vi "Gas Rack Cal UI.vi"(11 "Calling VI Ref":refnum<vi>) -> ()   [LabVIEW 2013]
uses:
  Type Defs/Units Type Def (DAQ Rack).ctl
  Type Defs/Gas Rack Channel Type Def (RIO).ctl
  Type Defs/Targets Type Def.ctl
  Type Defs/Target Cluster Type Def.ctl
  Type Defs/Setpoint Cluster Type Def.ctl
  Type Defs/Rack Version Type Def.ctl
  Type Defs/Registered System.ctl
  Type Defs/System Type.ctl
  Type Defs/TCP Data Stream Mode (PC).ctl
  <vilib>/Utility/miscctls.llb/LVRowAndColumnTypeDef.ctl
  <vilib>/Utility/file.llb/Write To Spreadsheet File (string).vi
  <vilib>/Utility/file.llb/Read From Spreadsheet File (string).vi
  <userlib>/_OpenG.lib/array/array.llb/Remove Duplicates from 1D Array (DBL)__ogtk.vi
  <userlib>/_OpenG.lib/array/array.llb/Search 1D Array (String)__ogtk.vi
  <vilib>/ptbypt/NI_PtbyPt.lvlib
  <vilib>/Analysis/NI_AALPro.lvlib
  <resource>/objmgr/daqmx.rc
  <vilib>/Utility/config.llb/NI_LVConfig.lvlib
  <vilib>/FTP/NI_FTP.lvlib
panel:
  out "RIO Found":bool
  out "Lost Connection":bool
  in  "Stop Second Loop":bool
  out "a0":dbl format="%#.4g"
  out "a2":dbl format="%#.4g"
  out "a1":dbl format="%#.4g"
  out "a3":dbl format="%#.4g"
  out "a4":dbl format="%#.4g"
  in  "App Dir":path
  in  "Load Indicator Tab":enum32{"Page 1"}(tab)
  in  "Header Tab":enum32{"Page 1", "Page 2"}(tab)
  in  "Header OK":bool
  in  "Header Cancel":bool
  in  "Header Comments":string[][](table)=[[""], [""], [""]]
  in  "Cal Standards Table":string[][](table)=[["", ""], ["", ""], ["", ""], ["", ""], ["", ""]]
  in  "Sys Cal Table":string[][](table)=[["", ""], ["", ""], ["", ""], ["", ""], ["", ""]]
  in  "Header Table 1":string[][](table)=[[""], [""], [""], [""], [""], [""], [""], [""]]
  in  "Header Table 2":string[][](table)=[[""], [""], [""], [""], [""], [""], [""]]
  in  "debug":bool=TRUE
  in  "Output Tab":enum32{"Page 1", "Page 2"}(tab)
  out "Row":i32
  in  "Main Tab":enum32{"Page 1", "Page 2"}(tab)
  in  "Channel to Cal":T1
  in  "Transfer Cal":bool
  in  "Verify Tab":enum32{"Page 1", "Page 2"}(tab)
  out "Ver Reading":dbl=0.0016 caption="reading" format="%#.4g"
  in  "Hide Devs":bool
  in  "Auto":bool
  in  "Hide Cal Values":bool
  in  "Verify Edit":bool
  in  "Verify Table":string[][](table)=[["", "0", "0"], ["", "3", "3"], ["", "6", "6"], ["", "9", "9"], ["", "12", "12"], ["", "15", "15"], ["", "", ""], ["", "", ""], ["", "", ""], ["", "", ""]]
  in  "Verify Read":bool
  in  "ms":u32=1000
  in  "avg":i32=5
  in  "Save Cal":bool
  in  "Cancel Verify":bool
  in  "Cal Tab":enum32{"Apply", "Cal"}(tab)
  in  "Cancel Cal":bool
  in  "Apply Cal":bool
  in  "Confirm Cal Point":bool
  in  "Master Value":dbl caption="cal pt" format="%#.4g"
  out "Cal Reading":dbl=0.0016 caption="reading" format="%#.4g"
  in  "4th Point Cal":bool
  out "Reading Value 4":dbl caption="reading" format="%#.4g"
  in  "Cal Value 4":dbl caption="cal pt" format="%#.4g"
  in  "5th Point Cal":bool
  out "Reading Value 5":dbl caption="reading" format="%#.4g"
  in  "Cal Value 5":dbl caption="cal pt" format="%#.4g"
  in  "Start Verification":bool
  in  "Header":bool
  out "Cal Table":string[][](table)=[["AI-00", "V", "", "", "", "", "", "", "", "", "", "", "", "", "", "", "", "", "", "", "", "", "", "", "", "", "", "", "", "", "", ""], ["AI-01", "V", "", "", "", "", "", "", "", "", "", "", "", "", "", "", "", "", "", "", "", "", "", "", "", "", "", "", "", "", "", ""], ["AI-02", "V", "", "", "", "", "", "", "", "", "", "", "", "", "", "", "", "", "", "", "", "", "", "", "", "", "", "", "", "", "", ""], ["AI-03", "V", "", "", "", "", "", "", "", "", "", "", "", "", "", "", "", "", "", "", "", "", "", "", "", "", "", "", "", "", "", ""], ["AI-04", "V", "", "", "", "", "", "", "", "", "", "", "", "", "", "", "", "", "", "", "", "", "", "", "", "", "", "", "", "", "", ""], ["AI-05", "V", "", "", "", "", "", "", "", "", "", "", "", "", "", "", "", "", "", "", "", "", "", "", "", "", "", "", "", "", "", ""], ["AI-06", "V", "", "", "", "", "", "", "", "", "", "", "", "", "", "", "", "", "", "", "", "", "", "", "", "", "", "", "", "", "", ""], ["AI-07", "V", "", "", "", "", "", "", "", "", "", "", "", "", "", "", "", "", "", "", "", "", "", "", "", "", "", "", "", "", "", ""], ["AI-08", "V", "", "", "", "", "", "", "", "", "", "", "", "", "", "", "", "", "", "", "", "", "", "", "", "", "", "", "", "", "", ""], ["AI-09", "V", "", "", "", "", "", "", "", "", "", "", "", "", "", "", "", "", "", "", "", "", "", "", "", "", "", "", "", "", "", ""], ["AI-10", "V", "", "", "", "", "", "", "", "", "", "", "", "", "", "", "", "", "", "", "", "", "", "", "", "", "", "", "", "", "", ""], ["AI-11", "V", "", "", "", "", "", "", "", "", "", "", "", "", "", "", "", "", "", "", "", "", "", "", "", "", "", "", "", "", "", ""], ["AI-12", "V", "", "", "", "", "", "", "", "", "", "", "", "", "", "", "", "", "", "", "", "", "", "", "", "", "", "", "", "", "", ""], ["AI-13", "V", "", "", "", "", "", "", "", "", "", "", "", "", "", "", "", "", "", "", "", "", "", "", "", "", "", "", "", "", "", ""], ["AI-14", "V", "", "", "", "", "", "", "", "", "", "", "", "", "", "", "", "", "", "", "", "", "", "", "", "", "", "", "", "", "", ""], ["AI-15", "V", "", "", "", "", "", "", "", "", "", "", "", "", "", "", "", "", "", "", "", "", "", "", "", "", "", "", "", "", "", ""], ["AI-16", "V", "", "", "", "", "", "", "", "", "", "", "", "", "", "", "", "", "", "", "", "", "", "", "", "", "", "", "", "", "", ""], ["AI-17", "V", "", "", "", "", "", "", "", "", "", "", "", "", "", "", "", "", "", "", "", "", "", "", "", "", "", "", "", "", "", ""], ["AI-18", "V", "", "", "", "", "", "", "", "", "", "", "", "", "", "", "", "", "", "", "", "", "", "", "", "", "", "", "", "", "", ""], ["AI-19", "V", "", "", "", "", "", "", "", "", "", "", "", "", "", "", "", "", "", "", "", "", "", "", "", "", "", "", "", "", "", ""], ["AI-20", "V", "", "", "", "", "", "", "", "", "", "", "", "", "", "", "", "", "", "", "", "", "", "", "", "", "", "", "", "", "", ""], ["AI-21", "V", "", "", "", "", "", "", "", "", "", "", "", "", "", "", "", "", "", "", "", "", "", "", "", "", "", "", "", "", "", ""], ["AI-22", "V", "", "", "", "", "", "", "", "", "", "", "", "", "", "", "", "", "", "", "", "", "", "", "", "", "", "", "", "", "", ""], ["AI-23", "V", "", "", "", "", "", "", "", "", "", "", "", "", "", "", "", "", "", "", "", "", "", "", "", "", "", "", "", "", "", ""], ["AI-24", "V", "", "", "", "", "", "", "", "", "", "", "", "", "", "", "", "", "", "", "", "", "", "", "", "", "", "", "", "", "", ""], ["AI-25", "V", "", "", "", "", "", "", "", "", "", "", "", "", "", "", "", "", "", "", "", "", "", "", "", "", "", "", "", "", "", ""], ["AI-26", "V", "", "", "", "", "", "", "", "", "", "", "", "", "", "", "", "", "", "", "", "", "", "", "", "", "", "", "", "", "", ""], ["AI-27", "V", "", "", "", "", "", "", "", "", "", "", "", "", "", "", "", "", "", "", "", "", "", "", "", "", "", "", "", "", "", ""], ["AI-28", "V", "", "", "", "", "", "", "", "", "", "", "", "", "", "", "", "", "", "", "", "", "", "", "", "", "", "", "", "", "", ""], ["AI-29", "V", "", "", "", "", "", "", "", "", "", "", "", "", "", "", "", "", "", "", "", "", "", "", "", "", "", "", "", "", "", ""], ["AI-30", "V", "", "", "", "", "", "", "", "", "", "", "", "", "", "", "", "", "", "", "", "", "", "", "", "", "", "", "", "", "", ""], ["AI-31", "V", "", "", "", "", "", "", "", "", "", "", "", "", "", "", "", "", "", "", "", "", "", "", "", "", "", "", "", "", "", ""], ["TC-00", "degF", "", "", "", "", "", "", "", "", "", "", "", "", "", "", "", "", "", "", "", "", "", "", "", "", "", "", "", "", "", ""], ["TC-01", "degF", "", "", "", "", "", "", "", "", "", "", "", "", "", "", "", "", "", "", "", "", "", "", "", "", "", "", "", "", "", ""], ["TC-02", "degF", "", "", "", "", "", "", "", "", "", "", "", "", "", "", "", "", "", "", "", "", "", "", "", "", "", "", "", "", "", ""], ["TC-03", "degF", "", "", "", "", "", "", "", "", "", "", "", "", "", "", "", "", "", "", "", "", "", "", "", "", "", "", "", "", "", ""], ["TC-04", "degF", "", "", "", "", "", "", "", "", "", "", "", "", "", "", "", "", "", "", "", "", "", "", "", "", "", "", "", "", "", ""], ["TC-05", "degF", "", "", "", "", "", "", "", "", "", "", "", "", "", "", "", "", "", "", "", "", "", "", "", "", "", "", "", "", "", ""], ["TC-06", "degF", "", "", "", "", "", "", "", "", "", "", "", "", "", "", "", "", "", "", "", "", "", "", "", "", "", "", "", "", "", ""], ["TC-07", "degF", "", "", "", "", "", "", "", "", "", "", "", "", "", "", "", "", "", "", "", "", "", "", "", "", "", "", "", "", "", ""], ["TC-08", "degF", "", "", "", "", "", "", "", "", "", "", "", "", "", "", "", "", "", "", "", "", "", "", "", "", "", "", "", "", "", ""], ["TC-09", "degF", "", "", "", "", "", "", "", "", "", "", "", "", "", "", "", "", "", "", "", "", "", "", "", "", "", "", "", "", "", ""], ["TC-10", "degF", "", "", "", "", "", "", "", "", "", "", "", "", "", "", "", "", "", "", "", "", "", "", "", "", "", "", "", "", "", ""], ["TC-11", "degF", "", "", "", "", "", "", "", "", "", "", "", "", "", "", "", "", "", "", "", "", "", "", "", "", "", "", "", "", "", ""], ["TC-12", "degF", "", "", "", "", "", "", "", "", "", "", "", "", "", "", "", "", "", "", "", "", "", "", "", "", "", "", "", "", "", ""], ["TC-13", "degF", "", "", "", "", "", "", "", "", "", "", "", "", "", "", "", "", "", "", "", "", "", "", "", "", "", "", "", "", "", ""], ["TC-14", "degF", "", "", "", "", "", "", "", "", "", "", "", "", "", "", "", "", "", "", "", "", "", "", "", "", "", "", "", "", "", ""], ["TC-15", "degF", "", "", "", "", "", "", "", "", "", "", "", "", "", "", "", "", "", "", "", "", "", "", "", "", "", "", "", "", "", ""], ["", "", "", "", "", "", "", "", "", "", "", "", "", "", "", "", "", "", "", "", "", "", "", "", "", "", "", "", "", "", "", ""]]
  out "Tank IP:":string
  in  "Start Cal":bool
  in  "1st Point Cal":bool
  out "Reading Value 1":dbl caption="Read Data" format="%#.4g"
  in  "Cal Value 1":dbl caption="Cal Point" format="%#.4g"
  in  "2nd Point Cal":bool
  out "Reading Value 2":dbl caption="reading" format="%#.4g"
  in  "Cal Value 2":dbl caption="cal pt" format="%#.4g"
  in  "Cal Unit":T2
  in  "3rd Point Cal":bool
  out "Reading Value 3":dbl caption="reading" format="%#.4g"
  in  "Cal Value 3":dbl caption="cal pt" format="%#.4g"
  in  "View Spreadsheet":bool
  # "Channel Data"
  # "System Calibration Components"
  # "Calibration Standards Used"
  # "Output Control"
  # "Enter Header Info"
  # "Calibration"
  # "Verification"
  # "Select Channel to Calibrate"
  # "Cal Spreadsheet"
  # "*Excel must be closed to return control to this app."
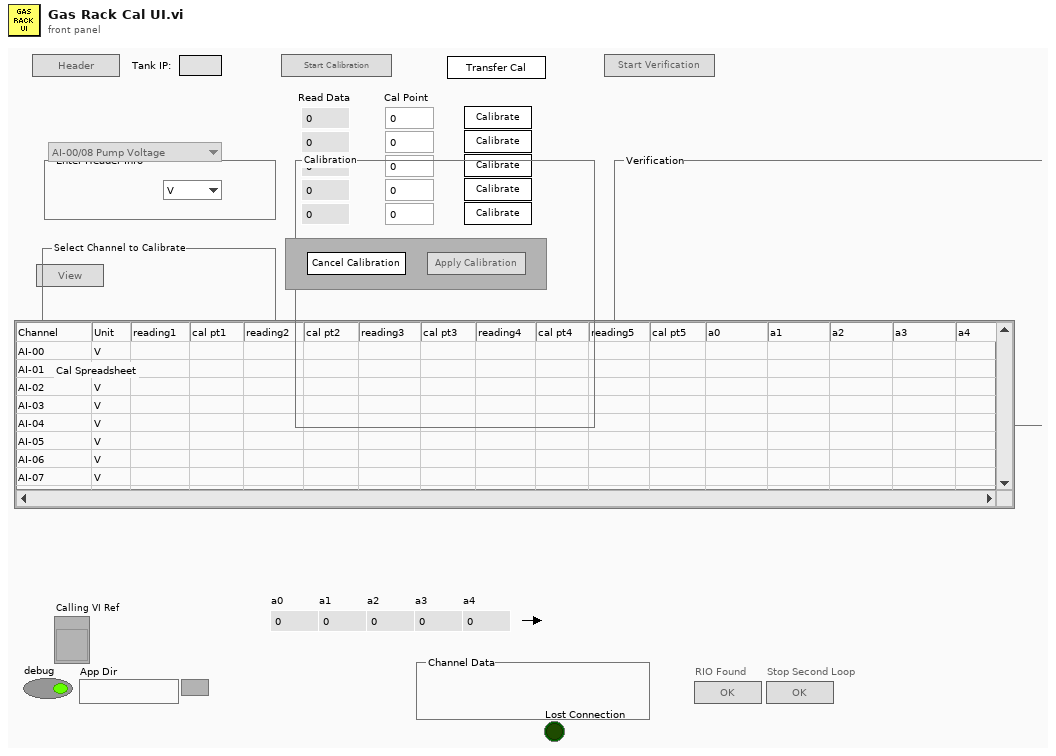
[diagram p1: front panel]
types:
  T1 = typedef "Gas Rack Channel Type Def (RIO).ctl" = enum16{"AI-00/08 Pump Voltage", "AI-01/09 Pump Current", "AI-02/10 Pressure", "AI-03/11 Flow", "AI-04/12 Controller Voltage", "AI-07/15 Controller Current", "AI-06/14 Temperature", "AI-05/13 Spare"}
  T2 = typedef "Units Type Def (DAQ Rack).ctl" = enum16{"V", "mA", "A", "Hz", "deg C"}
  T3 = typedef "Registered System.ctl" = cluster{"System Type":T4, "Serial Number":string, "ID":string, "Cal File?":bool}
  T4 = typedef "System Type.ctl" = enum16{"DAQ Rack", "DAQ Cart", "RIO", "cDAQ", "unknown", "open"}
  T5 = typedef "Rack Version Type Def.ctl" = enum16{"Volts & TC", "Volts", "RIO", "cDAQ", "Volts & Current", "Cart"}
  T6 = typedef "Targets Type Def.ctl" = cluster{"V Targets":T7, "5V Targets":T7, "mA Targets":T7, "A Targets":T7, "Hz Targets":T7, "TC Targets":T7, "V Setpoints":T8, "5V Setpoints":T8, "mA Setpoints ":T8, "A Setpoints":T8, "Hz Setpoints":T8, "25A Setpoints":T8, "25A Targets":T7, "CT Targets":T7, "DegC Targets":T7, "kPa Targets":T7, "LpH Targets":T7, "CT Setpoints":T8, "DegC Setpoints":T8, "kPa Setpoints":T8, "LpH Setpoints":T8}
  T7 = typedef "Target Cluster Type Def.ctl" = cluster{"target1":dbl, "target2":dbl, "target3":dbl, "target4":dbl, "target5":dbl, "target6":dbl, "target7":dbl, "target8":dbl, "target9":dbl, "target10":dbl}
  T8 = typedef "Setpoint Cluster Type Def.ctl" = cluster{"setpoint1":dbl, "setpoint2":dbl, "setpoint3":dbl, "setpoint4":dbl, "setpoint5":dbl}
  T9 = cluster{"Error":errorcluster, "Cal Log":string[][], "Cal Log Header":string[], "Cal Files Base Path":path, "Default Cal Log":string[][], "Samples to Avg":i32, "Base Path":path, "Cal Targets Path":path, "Calling VI Ref":refnum<vi>, "Selected Chassis":tag, "debug":bool, "Verify Table":string[][], "Cal Template Path":path, "Cal Spreadsheet Path":path, "Verify Table Ref":refnum<vi>, "Init Mean":bool, "Auto":bool, "App Dir":path, "DAQ Rack":string, "Cal File Path":path, "Targets":T6, "Cal Unit":T2, "Channel to Cal":T1, "Rack Version":T5, "Verification":bool, "Registered Systems":T3[], "Desired System":T3, "Cal Target Array":string[], "LastCalPt":i32, "StreamCtrlActive":bool}
  T10 = enum8{"Enabled", "Disabled", "Disabled and Grayed Out"}
  T11 = typedef "TCP Data Stream Mode (PC).ctl" = enum16{"Init", "Read Data", "Close"}
  T12 = typedef "LVRowAndColumnTypeDef.ctl" = cluster{"Row":i32, "Column":i32}
  T13 = enum32{"Bad", "Idle", "Run top level", "Running"}
  T14 = cluster{"[0]":dbl, "[1]":dbl, "[2]":dbl, "[3]":dbl, "[4]":dbl, "[5]":dbl, "[6]":dbl, "[7]":dbl, "[8]":dbl, "[9]":dbl}
  T15 = typedef "NI_LVConfig.lvlib/Config Data RefNum.ctl" = refnum<k1>
  T16 = typedef "New Channel Type Def (RIO).ctl" = enum16{"AI-00/08 Pos 1 Pump Voltage", "AI-01/09 Pos 2 Pump Voltage", "AI-02/10 Pos 3 Pump Voltage", "AI-03/11 Pos 4 Pump Voltage", "AI-04/12 Pos 5 Pump Voltage", "AI-05/13 Pos 6 Pump Voltage", "AI-06 Spare", "AI-14 Spare", "AI-07 Spare", "AI-15 Power Supply Voltage", "AI-16 Pos 1 Pump Current", "AI-17 Pos 2 Pump Current", "AI-18 Pos 3 Pump Current", "AI-19 Pos 4 Pump Current", "AI-20 Pos 5 Pump Current", "AI-21 Pos 6 Pump Current", "AI-16 Pos 1 Pump Speed", "AI-17 Pos 2 Pump Speed", "AI-18 Pos 3 Pump Speed", "AI-19 Pos 4 Pump Speed", "AI-20 Pos 5 Pump Speed", "AI-21 Pos 6 Pump Speed", "AI-22 Pos 1 Controller Current", "AI-23 Pos 2 Controller Current", "AI-24 Pos 3 Controller Current", "AI-25 Pos 4 Controller Current", "AI-26 Pos 5 Controller Current", "AI-27 Pos 6 Controller Current", "AI-28 Tank 1 Temperature", "AI-29 Tank 2 Temperature", "AI-30 Pos 1 Pump Pressure", "AI-31 Pos 2 Pump Pressure", "AI-32 Pos 3 Pump Pressure", "AI-33 Pos 4 Pump Pressure", "AI-34 Pos 5 Pump Pressure", "AI-35 Pos 6 Pump Pressure", "AI-36 Pos 1 Pump Flow", "AI-37 Pos 2 Pump Flow", "AI-38 Pos 3 Pump Flow", "AI-39 Pos 4 Pump Flow", "AI-40 Pos 5 Pump Flow", "AI-41 Pos 6 Pump Flow", "AI-42 Spare", "AI-43 Spare", "AI-44 Spare", "AI-45 Spare", "AI-46 Spare", "AI-47 Spare", "AI-00/08 Pos 1 Controller Voltage", "AI-01/09 Pos 2 Controller Voltage", "AI-02/10 Pos 3 Controller Voltage", "AI-03/11 Pos 4 Controller Voltage", "AI-04/12 Pos 5 Controller Voltage", "AI-05/13 Pos 6 Controller Voltage"}
  T17 = typedef "Rack Version Type Def.ctl" = enum16{"Volts & TC", "Volts", "RIO", "Volts & Current", "Cart"}
  T18 = typedef "Registered System.ctl" = cluster{"System Type":T19, "Serial Number":u32, "ID":string, "Cal File?":bool}
  T19 = typedef "System Type.ctl" = enum16{"DAQ Rack", "DAQ Cart", "RIO", "unknown", "open"}
  T20 = cluster{"Error":errorcluster, "Cal Log":string[][], "Cal Log Header":string[], "Cal Files Base Path":path, "Default Cal Log":string[][], "Samples to Avg":i32, "Base Path":path, "Cal Targets Path":path, "Calling VI Ref":refnum<vi>, "Selected Chassis":tag, "debug":bool, "Verify Table":string[][], "Cal Template Path":path, "Cal Spreadsheet Path":path, "Verify Table Ref":refnum<vi>, "Init Mean":bool, "Auto":bool, "App Dir":path, "DAQ Rack":string, "Cal File Path":path, "Targets":T6, "Cal Unit":T2, "Channel to Cal":T16, "Rack Version":T17, "Verification":bool, "Registered Systems":T18[], "Desired System":T18, "Cal Target Array":string[], "LastCalPt":i32}
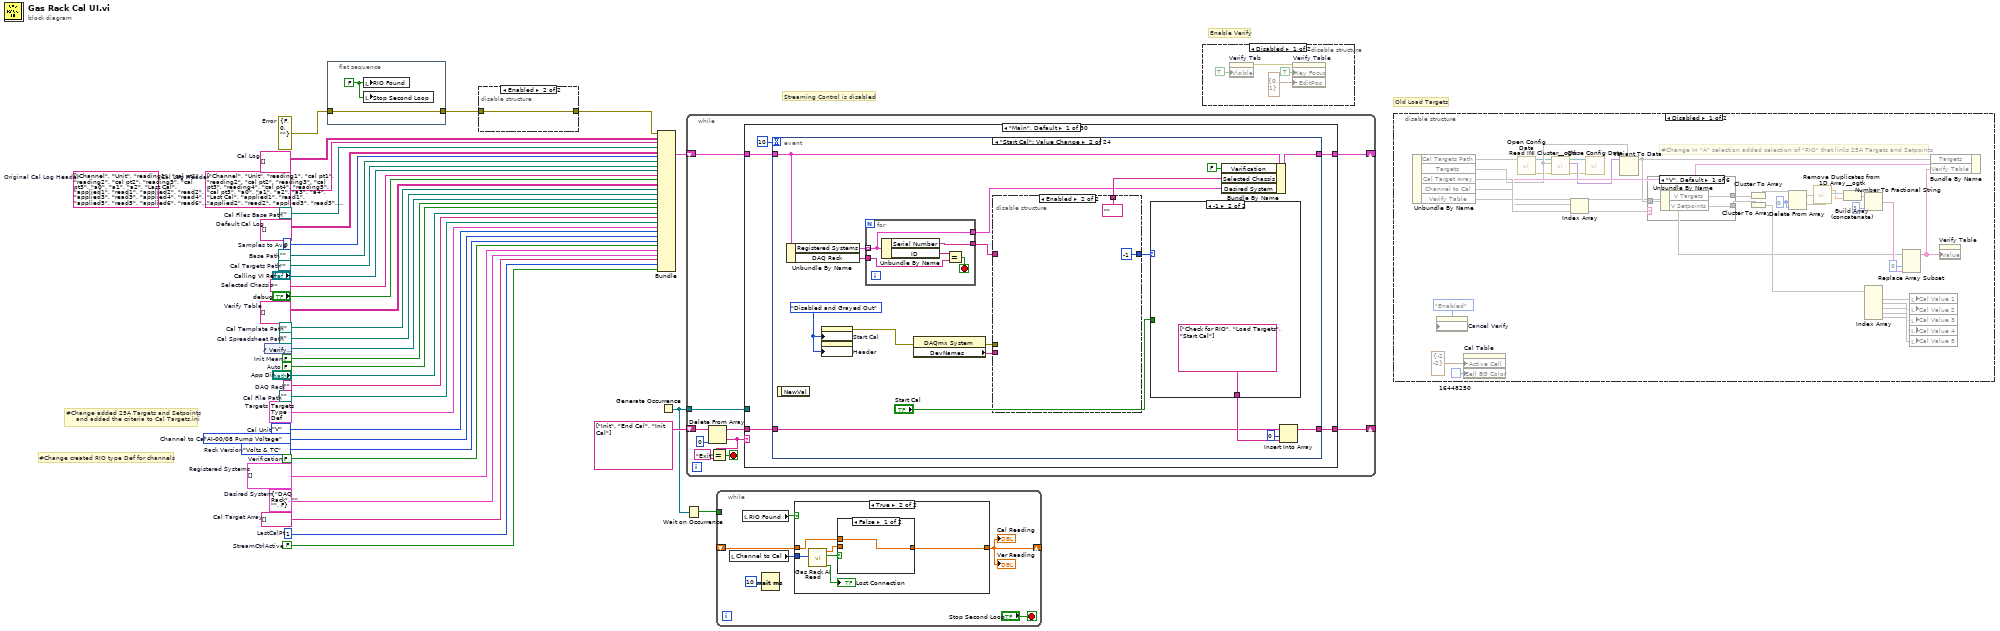
[diagram p0: block diagram]
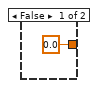
[diagram p2: hidden frame]
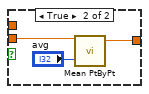
[diagram p3: hidden frame]
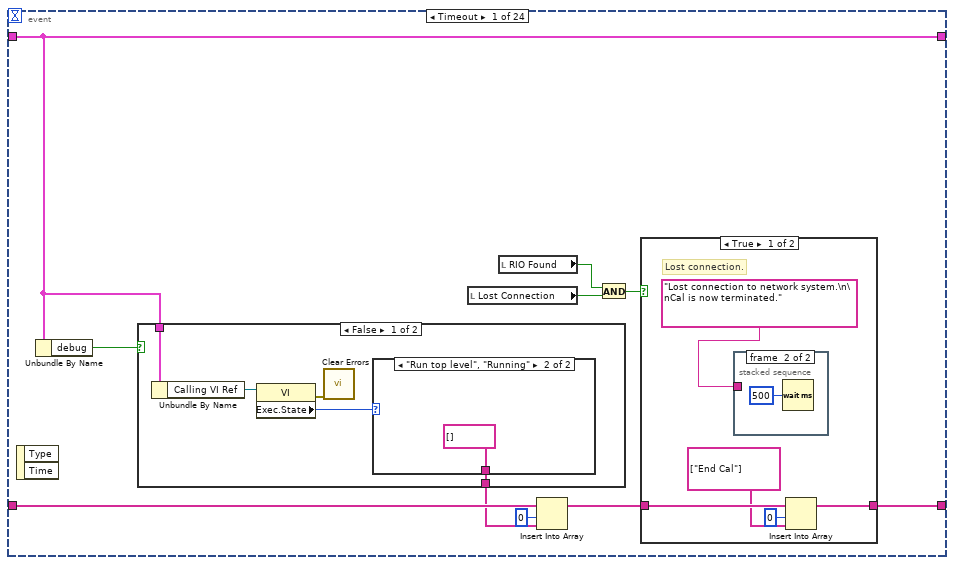
[diagram p4: hidden frame]
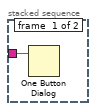
[diagram p5: hidden frame]
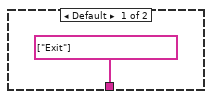
[diagram p7: hidden frame]
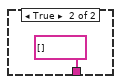
[diagram p8: hidden frame]
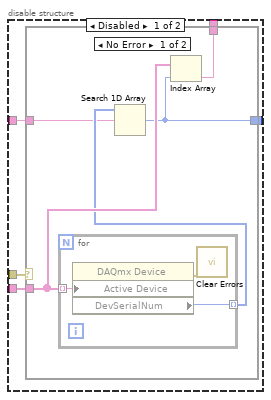
[diagram p9: hidden frame]
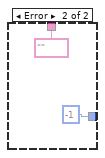
[diagram p10: hidden frame]
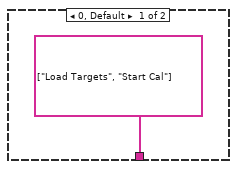
[diagram p11: hidden frame]
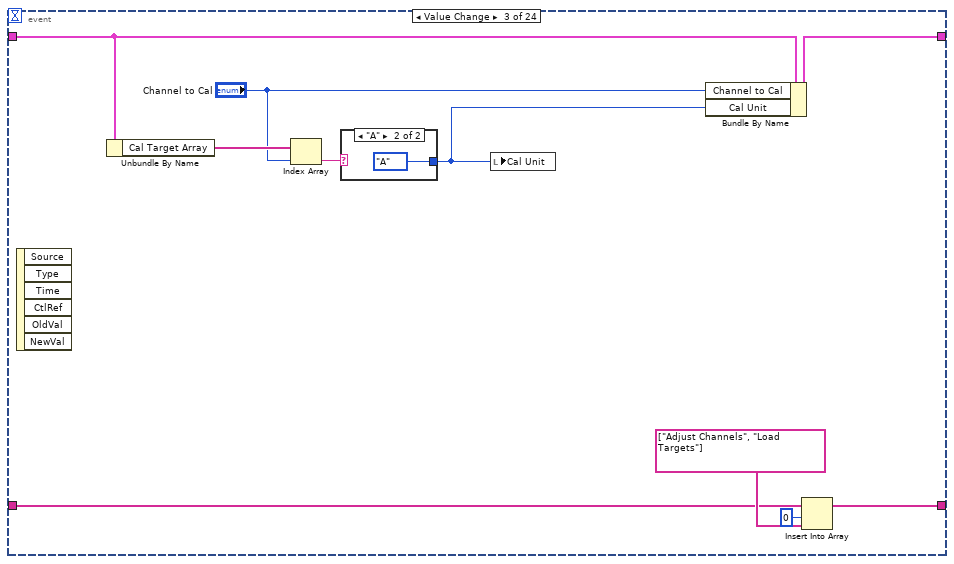
[diagram p12: hidden frame]
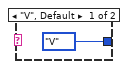
[diagram p13: hidden frame]
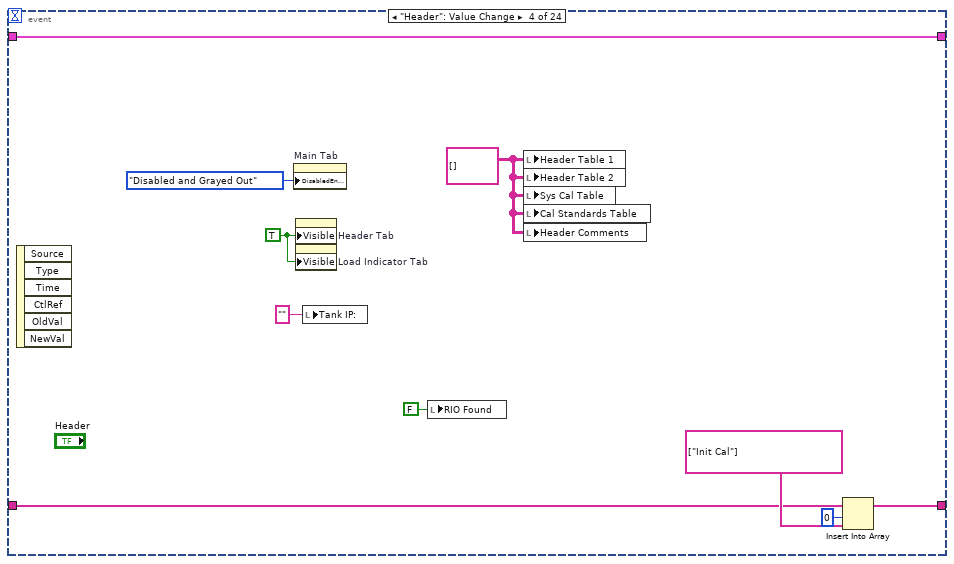
[diagram p14: hidden frame]
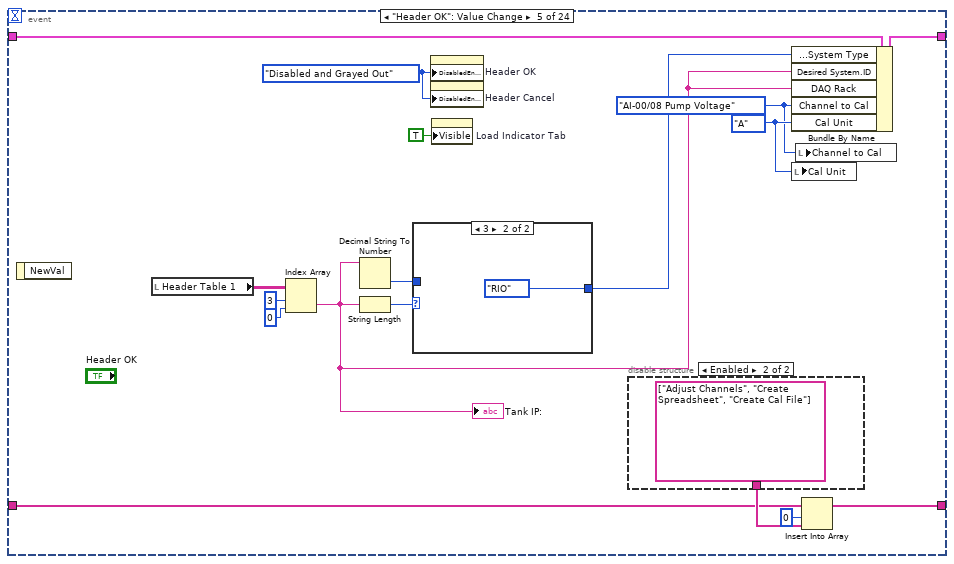
[diagram p15: hidden frame]
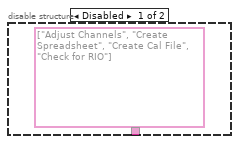
[diagram p16: hidden frame]
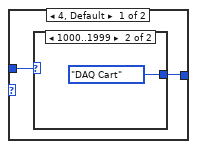
[diagram p17: hidden frame]
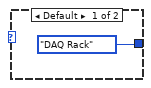
[diagram p18: hidden frame]
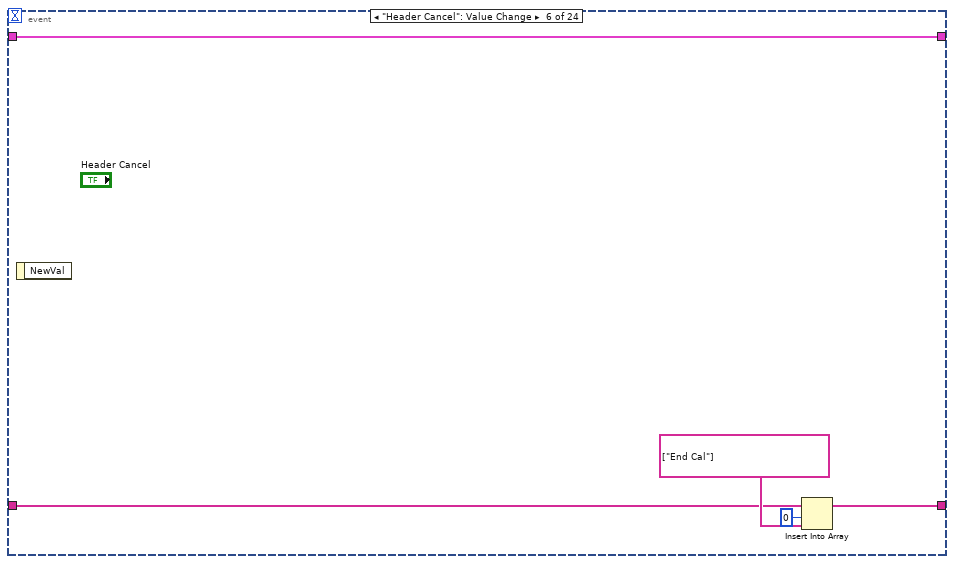
[diagram p19: hidden frame]
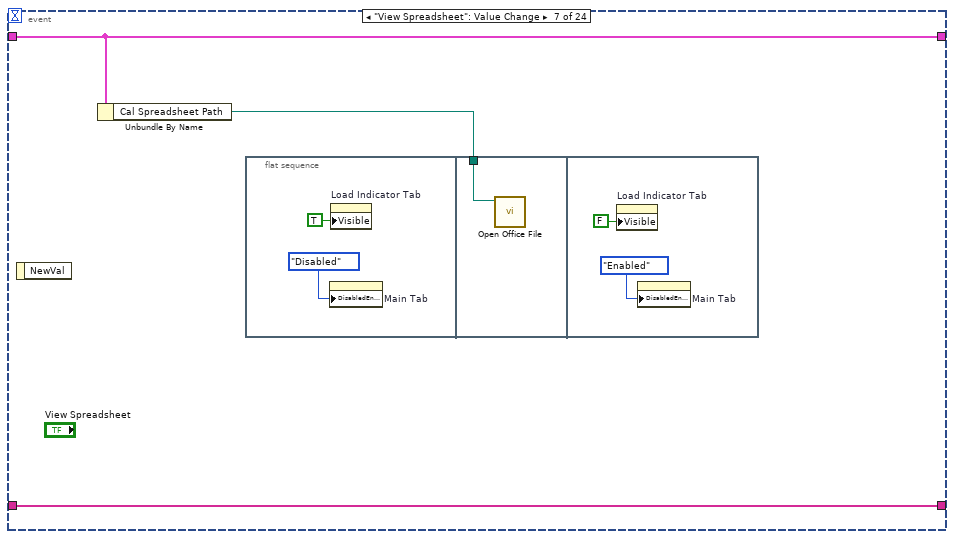
[diagram p20: hidden frame]
diagram:
  w1 = Gas_Rack_Channel_Type_Def_(RIO)."AI-00/08 Pump Voltage"  # Channel to Cal
  w8 = FALSE  # StreamCtrlActive
  w9 = 1  # LastCalPt
  w11 = string[] ["Channel", "Unit", "reading1", "cal pt1", "reading2", "cal pt2", "reading3", "cal pt3", "reading4", "cal pt4", "reading5", "cal pt5", "a0", "a1", "a2", "a3", "a4", "Last Cal", "applied1", "read1", "applied2", "read2", "applied3", "read3", "applied4", "read4", "applied5", "read5", "applied6", "read6", "applied7", "read7", "applied8", "read8", "applied9", "read9", "applied10", "read10"]  # Cal Log Header
  w12 = string[] []  # Cal Target Array
  w13 = T3 {"System Type"=enum."DAQ Rack", "Serial Number"="", "ID"="", "Cal File?"=FALSE}  # Desired System
  w14 = T3[] []  # Registered Systems
  w15 = FALSE  # Verification
  w16 = Rack_Version_Type_Def."Volts & TC"  # Rack Version
  w17 = Units_Type_Def_(DAQ_Rack)."V"  # Cal Unit
  w18 = T6 {"V Targets"={"target1"=0.0, "target2"=0.0, "target3"=0.0, "target4"=0.0, "target5"=0.0, "target6"=0.0, "target7"=0.0, "target8"=0.0, "target9"=0.0, "target10"=0.0}, "5V Targets"={"target1"=0.0, "target2"=0.0, "target3"=0.0, "target4"=0.0, "target5"=0.0, "target6"=0.0, "target7"=0.0, "target8"=0.0, "target9"=0.0, "target10"=0.0}, "mA Targets"={"target1"=0.0, "target2"=0.0, "target3"=0.0, "target4"=0.0, "target5"=0.0, "target6"=0.0, "target7"=0.0, "target8"=0.0, "target9"=1.0, "target10"=0.0}, "A Targets"={"target1"=0.0, "target2"=0.0, "target3"=0.0, "target4"=0.0, "target5"=0.0, "target6"=0.0, "target7"=0.0, "target8"=0.0, "target9"=0.0, "target10"=0.0}, "Hz Targets"={"target1"=0.0, "target2"=0.0, "target3"=0.0, "target4"=0.0, "target5"=0.0, "target6"=0.0, "target7"=0.0, "target8"=0.0, "target9"=0.0, "target10"=0.0}, "TC Targets"={"target1"=0.0, "target2"=0.0, "target3"=0.0, "target4"=0.0, "target5"=0.0, "target6"=0.0, "target7"=0.0, "target8"=0.0, "target9"=0.0, "target10"=0.0}, "V Setpoints"={"setpoint1"=0.0, "setpoint2"=0.0, "setpoint3"=0.0, "setpoint4"=0.0, "setpoint5"=0.0}, "5V Setpoints"={"setpoint1"=0.0, "setpoint2"=0.0, "setpoint3"=0.0, "setpoint4"=0.0, "setpoint5"=0.0}, "mA Setpoints "={"setpoint1"=0.0, "setpoint2"=0.0, "setpoint3"=0.0, "setpoint4"=0.0, "setpoint5"=0.0}, "A Setpoints"={"setpoint1"=0.0, "setpoint2"=0.0, "setpoint3"=0.0, "setpoint4"=0.0, "setpoint5"=0.0}, "Hz Setpoints"={"setpoint1"=0.0, "setpoint2"=0.0, "setpoint3"=0.0, "setpoint4"=0.0, "setpoint5"=0.0}, "25A Setpoints"={"setpoint1"=0.0, "setpoint2"=0.0, "setpoint3"=0.0, "setpoint4"=0.0, "setpoint5"=0.0}, "25A Targets"={"target1"=0.0, "target2"=0.0, "target3"=0.0, "target4"=0.0, "target5"=0.0, "target6"=0.0, "target7"=0.0, "target8"=0.0, "target9"=0.0, "target10"=0.0}, "CT Targets"={"target1"=0.0, "target2"=0.0, "target3"=0.0, "target4"=0.0, "target5"=0.0, "target6"=0.0, "target7"=0.0, "target8"=0.0, "target9"=0.0, "target10"=0.0}, "DegC Targets"={"target1"=0.0, "target2"=0.0, "target3"=0.0, "target4"=0.0, "target5"=0.0, "target6"=0.0, "target7"=0.0, "target8"=0.0, "target9"=0.0, "target10"=0.0}, "kPa Targets"={"target1"=0.0, "target2"=0.0, "target3"=0.0, "target4"=0.0, "target5"=0.0, "target6"=0.0, "target7"=0.0, "target8"=0.0, "target9"=0.0, "target10"=0.0}, "LpH Targets"={"target1"=0.0, "target2"=0.0, "target3"=0.0, "target4"=0.0, "target5"=0.0, "target6"=0.0, "target7"=0.0, "target8"=0.0, "target9"=0.0, "target10"=0.0}, "CT Setpoints"={"setpoint1"=0.0, "setpoint2"=0.0, "setpoint3"=0.0, "setpoint4"=0.0, "setpoint5"=0.0}, "DegC Setpoints"={"setpoint1"=0.0, "setpoint2"=0.0, "setpoint3"=0.0, "setpoint4"=0.0, "setpoint5"=0.0}, "kPa Setpoints"={"setpoint1"=0.0, "setpoint2"=0.0, "setpoint3"=0.0, "setpoint4"=0.0, "setpoint5"=0.0}, "LpH Setpoints"={"setpoint1"=0.0, "setpoint2"=0.0, "setpoint3"=0.0, "setpoint4"=0.0, "setpoint5"=0.0}}  # Targets
  w19 = path ""  # Cal File Path
  w20 = ""  # DAQ Rack
  w22 = FALSE  # Auto
  w23 = FALSE  # Init Mean
  w25 = path ""  # Cal Spreadsheet Path
  w26 = path ""  # Cal Template Path
  w27 = string[][] []  # Verify Table
  w29 = tag ""  # Selected Chassis
  w31 = path ""  # Cal Targets Path
  w32 = path ""  # Base Path
  w33 = 0  # Samples to Avg
  w34 = string[][] []  # Default Cal Log
  w35 = path ""  # Cal Files Base Path
  (unwired) string[] ["Channel", "Unit", "reading1", "cal pt1", "reading2", "cal pt2", "reading3", "cal pt3", "a0", "a1", "a2", "Last Cal", "applied1", "read1", "applied2", "read2", "applied3", "read3", "applied4", "read4", "applied5", "read5", "applied6", "read6", "applied7", "read7", "applied8", "read8", "applied9", "read9", "applied10", "read10"]  # Original Cal Log Header
  w36 = string[][] []  # Cal Log
  w10 = errorcluster {"status"=FALSE, "code"=0, "source"=""}  # Error
  # "Old Load Targets"
  # "Streaming Control is disabled"
  # "Enable Verify"
  # "#Change created RIO type Def for channels"
  # "#Change added 25A Targets and Setpoints\n     and added the criteria to Cal Targets.ini"
  n1 = control-ref of="Verify Table Ref"() -> (w24:refnum<vi>)
  n2 = flat-sequence {
    tunnel: w10 -> [w38]
    tunnel: [w38] -> w7
    frame #0 {
      w37 = FALSE ("RIO Found")
      n3 = local write "RIO Found"(w37) -> ()
      n4 = local write "Stop Second Loop"(w37) -> ()
    }
  }
  n5 = disable-structure shown="Enabled" {
    disable-tunnel: w7 -> [w42 w43]
    disable-tunnel: [w40 w43] -> w6
    frame Disabled {
      w39 = TRUE ("Visible")
      n6 = property on="Cal Tab" class="TabCtl (strict)"(error in=w42, "Visible"=w39) -> (error out=w41:errorcluster)  [unwired: 1 in, 1 out]
      n7 = property on="Verify Tab" class="TabCtl (strict)"(error in=w41, "Visible"=w39) -> (error out=w40:errorcluster)  [unwired: 1 in, 1 out]
    }
    frame Enabled {
    }
  }
  n8 = Bundle("Error"=w6, "Cal Log"=w36, "Cal Log Header"=w11, "Cal Files Base Path"=w35, "Default Cal Log"=w34, "Samples to Avg"=w33, "Base Path"=w32, "Cal Targets Path"=w31, "Calling VI Ref"="Calling VI Ref", "Selected Chassis"=w29, "debug"="debug", "Verify Table"=w27, "Cal Template Path"=w26, "Cal Spreadsheet Path"=w25, "Verify Table Ref"=w24, "Init Mean"=w23, "Auto"=w22, "App Dir"="App Dir", "DAQ Rack"=w20, "Cal File Path"=w19, "Targets"=w18, "Cal Unit"=w17, "Channel to Cal"=w1, "Rack Version"=w16, "Verification"=w15, "Registered Systems"=w14, "Desired System"=w13, "Cal Target Array"=w12, "LastCalPt"=w9, "StreamCtrlActive"=w8) -> (w4:T9)  [unwired: 1 in]
  n9 = Generate Occurrence() -> (w3:refnum<k4>)
  n10 = Wait on Occurrence(2:w3) -> (0:w2:bool)  [unwired: 2 in]
  n11 = while {
    shift-right: [w46] -> _
    shift-left: string[] ["Init", "End Cal", "Init Cal"] -> [w53]
    shift-right: [w48] -> _
    shift-left: w4 -> [w49]
    tunnel: w3 -> [w44]
    stop <- w52 stop-if-true
    n12 = Delete From Array(array=w53, index=0) -> (deleted portion=w45:string, array with subset deleted=w51:string[])  [unwired: 1 in]
    n13 = Equal?(x=w45, y="Exit" ("x")) -> (x = y?=w52:bool)
    n14 = case shown="\"Main\", Default" w45 {
      selector: w45 -> [_ _ _ _ _ _ _ _ _ _ _ _ _ _ _ w859 _ _ _ _ _ _ _ _ _ _ _ _ _ _]
      tunnel: w51 -> [w57 w432 w447 w455 w472 w521 w551 w554 w558 w589 w618 w647 w671 w729 w849 w861 w875 w891 w975 w1002 w1012 w1075 w1153 w1176 w1193 w1204 w1227 w1240 w1248 w1251]
      tunnel: w49 -> [w56 w425 w448 w461 w469 w520 w550 w553 w556 w592 w620 w641 w669 w777 w852 w856 w876 w885 w961 w986 w1013 w1036 w1114 w1175 w1191 w1202 w1224 w1230 w1246 w1250]
      tunnel: [w55 w409 w448 w460 w469 w519 w549 w553 w556 w591 w620 w640 w673 w786 w852 w855 w876 w885 w961 w981 w1013 w1036 w1114 w1175 w1190 w1202 w1224 w1230 w1247 w1250] -> w48
      tunnel: [w54 w432 w447 w452 w471 w521 w551 w554 w557 w590 w619 w648 w672 w728 w849 w861 w875 w892 w974 w1003 w1012 w1076 w1154 w1176 w1192 w1203 w1227 w1241 w1248 w1251] -> w46
      tunnel: w44 -> [_ w408 _ _ _ _ _ _ _ _ _ _ _ _ _ _ _ _ _ _ _ _ _ _ _ _ _ _ _ _]
      frame "Main", Default {
        n15 = event shown="[1] \"Start Cal\": Value Change" {
          selector: _ -> [_ _ _ _ _ _ _ _ _ _ _ _ _ _ _ _ _ _ _ _ _ _ _ _]
          dyn-events: _ -> [_ _ _ _ _ _ _ _ _ _ _ _ _ _ _ _ _ _ _ _ _ _ _ _]
          timeout: 10 -> [_ _ _ _ _ _ _ _ _ _ _ _ _ _ _ _ _ _ _ _ _ _ _ _]
          tunnel: w57 -> [w68 w100 w133 w143 w161 w176 w180 _ _ _ _ _ _ w239 w264 _ w307 _ w326 w359 w365 w389 w396 w402]
          tunnel: [w66 w96 w136 w148 w155 w174 w178 w193 w201 w209 w217 w225 w228 w242 w266 w301 w305 w314 w327 w360 w363 w382 w398 w403] -> w55
          tunnel: w56 -> [w66 w97 w131 w148 w156 w174 w178 w193 w201 w209 w217 w225 w228 w244 w266 w301 w306 w315 w327 w360 w363 w382 w398 w404]
          tunnel: [w61 w101 w132 w142 w162 w175 w180 w190 w198 w206 w214 w222 string[] ["Stop Verification"] w240 w264 string[] ["Save Cal"] w307 string[] ["Calc Dev", "Cal Review"] w326 w358 w364 w389 w397 w402] -> w54
          event Timeout {
            n16 = event-data() -> ()  [unwired: 1 in, 2 out]
            n17 = Unbundle By Name(w66) -> ("debug"=w65:bool)
            n18 = case shown="False" w65 {
              tunnel: [w81 string[] []] -> w67
              tunnel: w66 -> [w78 _]
              frame False {
                n19 = Unbundle By Name(w78) -> ("Calling VI Ref"=w80:refnum<vi>)
                n20 = property class="VI"(reference=w80) -> (error out=w77:errorcluster, "Exec.State"=w79:T13)  [unwired: 1 in, 1 out]
                n21 = call <vilib>:"Clear Errors.vi"("error in (no error)"=w77) -> ()  [unwired: 6 in, 1 out]
                n22 = case shown="\"Run top level\", \"Running\"" w79 {
                  tunnel: [string[] ["Exit"] string[] []] -> w81
                  frame Default {
                  }
                  frame "Run top level", "Running" {
                  }
                }
              }
              frame True {
              }
            }
            n23 = local read "Lost Connection"() -> (w60:bool)
            n24 = local read "RIO Found"() -> (w63:bool)
            n25 = Insert Into Array(array=w68, index=0, new element=w67) -> (w62:string[])
            n26 = And(x=w63, y=w60) -> (x .and. y?=w59:bool)
            n27 = case shown="True" w59 {
              tunnel: w62 -> [w73 w76]
              tunnel: [w70 w76] -> w61
              frame True {
                # "Lost connection."
                n28 = stacked-sequence {
                  tunnel: "Lost connection to network system.\n\nCal is now terminated." ("message") -> [w74 _]
                  frame #0 {
                    n29 = One Button Dialog(message=w74) -> ()  [unwired: 1 in, 1 out]
                  }
                  frame #1 {
                    n30 = Wait (ms)(milliseconds to wait=u32 500) -> ()  [unwired: 1 out]
                  }
                }
                n31 = Insert Into Array(array=w73, index=0, new element=string[] ["End Cal"]) -> (w70:string[])
              }
              frame False {
                # "Or not yet connected"
                # "Still connected."
              }
            }
          }
          event "Start Cal": Value Change {
            w92 = T10."Disabled and Grayed Out" ("Disabled")
            n32 = event-data() -> ()  [unwired: 1 in, 1 out]
            n33 = Unbundle By Name(w97) -> ("Registered Systems"=w89:T3[], "DAQ Rack"=w88:string)
            n34 = property on="Start Cal" class="Bool"("DisabledEnum"=w92) -> (error out=w91:errorcluster)  [unwired: 2 in, 1 out]
            n35 = property on="Header" class="Bool"("DisabledEnum"=w92) -> ()  [unwired: 2 in, 2 out]
            n36 = for {
              tunnel: w89 -> [w120] mode=indexing
              tunnel: w88 -> [w123]
              tunnel: [w121] -> w87
              tunnel: [w120] -> w86
              stop <- w122 stop-if-true
              n37 = Unbundle By Name(w120) -> ("Serial Number"=w121:string, "ID"=w124:string)
              n38 = Equal?(x=w124, y=w123) -> (x = y?=w122:bool)
            }
            n39 = property class="DAQmx System"(error in=w91) -> (error out=w94:errorcluster, "DevNames"=w99:tag[])  [unwired: 1 in, 1 out]
            n40 = disable-structure shown="Enabled" {
              disable-tunnel: w99 -> [w107 _]
              disable-tunnel: [w106 -1 ("index of element")] -> w98
              disable-tunnel: [w105 tag ""] -> w95
              disable-tunnel: w94 -> [w104 _]
              disable-tunnel: w87 -> [w103 _]
              frame Disabled {
                n41 = case shown="No Error" w104 {
                  tunnel: w103 -> [w108 _]
                  tunnel: w107 -> [w112 _]
                  tunnel: [w111 -1 ("index of element")] -> w106
                  tunnel: [w110 tag ""] -> w105
                  frame No Error {
                    n42 = for {
                      tunnel: w112 -> [w115] mode=indexing
                      tunnel: [w114] -> w109 mode=indexing
                      n43 = property class="DAQmx Device"("Active Device"=w115) -> (error out=w113:errorcluster, "DevSerialNum"=w114:u32)  [unwired: 2 in, 1 out]
                      n44 = call <vilib>:"Clear Errors.vi"("error in (no error)"=w113) -> ()  [unwired: 6 in, 1 out]
                    }
                    n45 = Search 1D Array(1D array=w109, element=w108) -> (index of element=w111:i32)  [unwired: 1 in]
                    n46 = Index Array(array=w112, index=w111) -> (element=w110:tag)
                  }
                  frame Error {
                  }
                }
              }
              frame Enabled {
              }
            }
            n47 = case shown="-1" w98 {
              tunnel: [string[] ["Load Targets", "Start Cal"] string[] ["Check for RIO", "Load Targets", "Start Cal"]] -> w102
              tunnel: "Start Cal" -> [_ _]
              frame 0, Default {
              }
              frame -1 {
              }
            }
            n48 = Bundle By Name(cluster=w97, "Verification"=FALSE, "Selected Chassis"=w95, "Desired System"=w86) -> (w96:T9)
            n49 = Insert Into Array(array=w100, index=0, new element=w102) -> (w101:string[])
          }
          event Value Change {
            n50 = event-data() -> ()  [unwired: 1 in, 6 out]
            n51 = Unbundle By Name(w131) -> ("Cal Target Array"=w130:string[])
            n52 = Index Array(array=w130, index="Channel to Cal") -> (element=w129:string)
            n53 = case shown="\"A\"" w129 {
              tunnel: [Units_Type_Def_(DAQ_Rack)."V" ("Cal Unit") Units_Type_Def_(DAQ_Rack)."A" ("Cal Unit")] -> w128
              frame "V", Default {
              }
              frame "A" {
              }
            }
            n54 = local write "Cal Unit"(w128) -> ()
            n55 = Bundle By Name(cluster=w131, "Channel to Cal"="Channel to Cal", "Cal Unit"=w128) -> (w136:T9)
            n56 = Insert Into Array(array=w133, index=0, new element=string[] ["Adjust Channels", "Load Targets"]) -> (w132:string[])
          }
          event "Header": Value Change {
            w146 = string[][] [] ("Header Table 1")
            w145 = TRUE ("Visible")
            n57 = event-data() -> ()  [unwired: 1 in, 6 out]
            n58 = property on="Main Tab" class="TabCtl (strict)"("DisabledEnum"=T10."Disabled and Grayed Out" ("Disabled")) -> ()  [unwired: 2 in, 2 out]
            n59 = property on="Header Tab" class="TabCtl (strict)"("Visible"=w145) -> ()  [unwired: 2 in, 2 out]
            n60 = property on="Load Indicator Tab" class="TabCtl (strict)"("Visible"=w145) -> ()  [unwired: 2 in, 2 out]
            n61 = local write "Tank IP:"("" ("DAQ Rack")) -> ()
            n62 = local write "RIO Found"(FALSE ("RIO Found")) -> ()
            n63 = local write "Header Table 1"(w146) -> ()
            n64 = local write "Header Table 2"(w146) -> ()
            n65 = local write "Sys Cal Table"(w146) -> ()
            n66 = local write "Cal Standards Table"(w146) -> ()
            n67 = local write "Header Comments"(w146) -> ()
            n68 = Insert Into Array(array=w143, index=0, new element=string[] ["Init Cal"]) -> (w142:string[])
          }
          event "Header OK": Value Change {
            w149 = Gas_Rack_Channel_Type_Def_(RIO)."AI-00/08 Pump Voltage" ("Channel to Cal")
            w154 = Units_Type_Def_(DAQ_Rack)."A" ("Cal Unit")
            w165 = T10."Disabled and Grayed Out" ("Disabled")
            n69 = event-data() -> ()  [unwired: 1 in, 1 out]
            n70 = local read "Header Table 1"() -> (w159:string[][])
            n71 = Index Array(array=w159, index (row)=3, index (col)=0 ("disabled index (col)")) -> (element=w151:string)
            "Tank IP:" <- w151
            n72 = Decimal String To Number(string=w151) -> (number=w150:i32)  [unwired: 2 in, 1 out]
            n73 = String Length(string=w151) -> (length=w153:i32)
            n74 = case shown="3" w153 {
              tunnel: [w168 System_Type."RIO" ("Desired System.System Type")] -> w152
              tunnel: w150 -> [w169 _]
              frame 4, Default {
                n75 = case shown="1000..1999" w169 {
                  tunnel: [System_Type."DAQ Rack" ("Desired System.System Type") System_Type."DAQ Cart" ("Desired System.System Type")] -> w168
                  frame Default {
                  }
                  frame 1000..1999 {
                  }
                }
              }
              frame 3 {
              }
            }
            n76 = property on="Header OK" class="Bool"("DisabledEnum"=w165) -> ()  [unwired: 2 in, 2 out]
            n77 = property on="Header Cancel" class="Bool"("DisabledEnum"=w165) -> ()  [unwired: 2 in, 2 out]
            n78 = property on="Load Indicator Tab" class="TabCtl (strict)"("Visible"=TRUE) -> ()  [unwired: 2 in, 2 out]
            n79 = disable-structure shown="Enabled" {
              disable-tunnel: [string[] ["Adjust Channels", "Create Spreadsheet", "Create Cal File", "Check for RIO"] string[] ["Adjust Channels", "Create Spreadsheet", "Create Cal File"]] -> w163
              frame Disabled {
              }
              frame Enabled {
              }
            }
            n80 = Bundle By Name(cluster=w156, "Desired System.System Type"=w152, "Desired System.ID"=w151, "DAQ Rack"=w151, "Channel to Cal"=w149, "Cal Unit"=w154) -> (w155:T9)
            n81 = local write "Cal Unit"(w154) -> ()
            n82 = local write "Channel to Cal"(w149) -> ()
            n83 = Insert Into Array(array=w161, index=0, new element=w163) -> (w162:string[])
          }
          event "Header Cancel": Value Change {
            n84 = event-data() -> ()  [unwired: 1 in, 1 out]
            n85 = Insert Into Array(array=w176, index=0, new element=string[] ["End Cal"]) -> (w175:string[])
          }
          event "View Spreadsheet": Value Change {
            n86 = event-data() -> ()  [unwired: 1 in, 1 out]
            n87 = Unbundle By Name(w178) -> ("Cal Spreadsheet Path"=w179:path)
            n88 = flat-sequence {
              tunnel: w179 -> [w183]
              frame #0 {
                n89 = property on="Main Tab" class="TabCtl (strict)"("DisabledEnum"=T10."Disabled" ("Disabled")) -> ()  [unwired: 2 in, 2 out]
                n90 = property on="Load Indicator Tab" class="TabCtl (strict)"("Visible"=TRUE) -> ()  [unwired: 2 in, 2 out]
              }
              frame #1 {
                n91 = call "Open Office File.vi"("Selection a Word (.doc, .docx), Excel (.xls, .xlsx), or Powerpoint (.ppt, .pptx) Document..."=w183) -> ()  [unwired: 10 in, 1 out]
              }
              frame #2 {
                n92 = property on="Load Indicator Tab" class="TabCtl (strict)"("Visible"=FALSE) -> ()  [unwired: 2 in, 2 out]
                n93 = property on="Main Tab" class="TabCtl (strict)"("DisabledEnum"=T10."Enabled" ("Disabled")) -> ()  [unwired: 2 in, 2 out]
              }
            }
          }
          event "1st Point Cal": Value Change {
            n94 = event-data() -> ()  [unwired: 1 in, 1 out]
            n95 = Select(t=T10."Disabled" ("Disabled"), s="1st Point Cal", f=T10."Enabled" ("Disabled")) -> (s? t:f=w189:T10)
            n96 = property on="Cal Value 1" class="DigNum (strict)"("DisabledEnum"=w189) -> ()  [unwired: 2 in, 2 out]
            n97 = property on="Cal Value 2" class="DigNum (strict)"("DisabledEnum"=w189) -> ()  [unwired: 2 in, 2 out]
            n98 = property on="Cal Value 3" class="DigNum (strict)"("DisabledEnum"=w189) -> ()  [unwired: 2 in, 2 out]
            n99 = property on="Cal Value 4" class="DigNum (strict)"("DisabledEnum"=w189) -> ()  [unwired: 2 in, 2 out]
            n100 = property on="Cal Value 5" class="DigNum (strict)"("DisabledEnum"=w189) -> ()  [unwired: 2 in, 2 out]
            n101 = property on="2nd Point Cal" class="Bool (strict)"("DisabledEnum"=w189) -> ()  [unwired: 2 in, 2 out]
            n102 = property on="3rd Point Cal" class="Bool (strict)"("DisabledEnum"=w189) -> ()  [unwired: 2 in, 2 out]
            n103 = property on="4th Point Cal" class="Bool (strict)"("DisabledEnum"=w189) -> ()  [unwired: 2 in, 2 out]
            n104 = property on="5th Point Cal" class="Bool (strict)"("DisabledEnum"=w189) -> ()  [unwired: 2 in, 2 out]
            n105 = Select(t=string[] ["Calibrating 1"], s="1st Point Cal", f=string[] ["Stop Calibrating"]) -> (s? t:f=w190:string[])
          }
          event "2nd Point Cal": Value Change {
            n106 = event-data() -> ()  [unwired: 1 in, 1 out]
            n107 = Select(t=T10."Disabled" ("Disabled"), s="2nd Point Cal", f=T10."Enabled" ("Disabled")) -> (s? t:f=w197:T10)
            n108 = property on="Cal Value 1" class="DigNum (strict)"("DisabledEnum"=w197) -> ()  [unwired: 2 in, 2 out]
            n109 = property on="Cal Value 2" class="DigNum (strict)"("DisabledEnum"=w197) -> ()  [unwired: 2 in, 2 out]
            n110 = property on="Cal Value 3" class="DigNum (strict)"("DisabledEnum"=w197) -> ()  [unwired: 2 in, 2 out]
            n111 = property on="Cal Value 4" class="DigNum (strict)"("DisabledEnum"=w197) -> ()  [unwired: 2 in, 2 out]
            n112 = property on="Cal Value 5" class="DigNum (strict)"("DisabledEnum"=w197) -> ()  [unwired: 2 in, 2 out]
            n113 = property on="1st Point Cal" class="Bool (strict)"("DisabledEnum"=w197) -> ()  [unwired: 2 in, 2 out]
            n114 = property on="3rd Point Cal" class="Bool (strict)"("DisabledEnum"=w197) -> ()  [unwired: 2 in, 2 out]
            n115 = property on="4th Point Cal" class="Bool (strict)"("DisabledEnum"=w197) -> ()  [unwired: 2 in, 2 out]
            n116 = property on="5th Point Cal" class="Bool (strict)"("DisabledEnum"=w197) -> ()  [unwired: 2 in, 2 out]
            n117 = Select(t=string[] ["Calibrating 2"], s="2nd Point Cal", f=string[] ["Stop Calibrating"]) -> (s? t:f=w198:string[])
          }
          event "3rd Point Cal": Value Change {
            n118 = event-data() -> ()  [unwired: 1 in, 1 out]
            n119 = Select(t=T10."Disabled" ("Disabled"), s="3rd Point Cal", f=T10."Enabled" ("Disabled")) -> (s? t:f=w205:T10)
            n120 = property on="Cal Value 1" class="DigNum (strict)"("DisabledEnum"=w205) -> ()  [unwired: 2 in, 2 out]
            n121 = property on="Cal Value 2" class="DigNum (strict)"("DisabledEnum"=w205) -> ()  [unwired: 2 in, 2 out]
            n122 = property on="Cal Value 3" class="DigNum (strict)"("DisabledEnum"=w205) -> ()  [unwired: 2 in, 2 out]
            n123 = property on="Cal Value 4" class="DigNum (strict)"("DisabledEnum"=w205) -> ()  [unwired: 2 in, 2 out]
            n124 = property on="Cal Value 5" class="DigNum (strict)"("DisabledEnum"=w205) -> ()  [unwired: 2 in, 2 out]
            n125 = property on="1st Point Cal" class="Bool (strict)"("DisabledEnum"=w205) -> ()  [unwired: 2 in, 2 out]
            n126 = property on="2nd Point Cal" class="Bool (strict)"("DisabledEnum"=w205) -> ()  [unwired: 2 in, 2 out]
            n127 = property on="4th Point Cal" class="Bool (strict)"("DisabledEnum"=w205) -> ()  [unwired: 2 in, 2 out]
            n128 = property on="5th Point Cal" class="Bool (strict)"("DisabledEnum"=w205) -> ()  [unwired: 2 in, 2 out]
            n129 = Select(t=string[] ["Calibrating 3"], s="3rd Point Cal", f=string[] ["Stop Calibrating"]) -> (s? t:f=w206:string[])
          }
          event "4th Point Cal": Value Change {
            n130 = event-data() -> ()  [unwired: 1 in, 6 out]
            n131 = Select(t=T10."Disabled" ("Disabled"), s="4th Point Cal", f=T10."Enabled" ("Disabled")) -> (s? t:f=w213:T10)
            n132 = property on="Cal Value 1" class="DigNum (strict)"("DisabledEnum"=w213) -> ()  [unwired: 2 in, 2 out]
            n133 = property on="Cal Value 2" class="DigNum (strict)"("DisabledEnum"=w213) -> ()  [unwired: 2 in, 2 out]
            n134 = property on="Cal Value 3" class="DigNum (strict)"("DisabledEnum"=w213) -> ()  [unwired: 2 in, 2 out]
            n135 = property on="Cal Value 4" class="DigNum (strict)"("DisabledEnum"=w213) -> ()  [unwired: 2 in, 2 out]
            n136 = property on="Cal Value 5" class="DigNum (strict)"("DisabledEnum"=w213) -> ()  [unwired: 2 in, 2 out]
            n137 = property on="1st Point Cal" class="Bool (strict)"("DisabledEnum"=w213) -> ()  [unwired: 2 in, 2 out]
            n138 = property on="2nd Point Cal" class="Bool (strict)"("DisabledEnum"=w213) -> ()  [unwired: 2 in, 2 out]
            n139 = property on="3rd Point Cal" class="Bool (strict)"("DisabledEnum"=w213) -> ()  [unwired: 2 in, 2 out]
            n140 = property on="5th Point Cal" class="Bool (strict)"("DisabledEnum"=w213) -> ()  [unwired: 2 in, 2 out]
            n141 = Select(t=string[] ["Calibrating 4"], s="4th Point Cal", f=string[] ["Stop Calibrating"]) -> (s? t:f=w214:string[])
          }
          event "5th Point Cal": Value Change {
            n142 = event-data() -> ()  [unwired: 1 in, 6 out]
            n143 = Select(t=T10."Disabled" ("Disabled"), s="5th Point Cal", f=T10."Enabled" ("Disabled")) -> (s? t:f=w221:T10)
            n144 = property on="Cal Value 1" class="DigNum (strict)"("DisabledEnum"=w221) -> ()  [unwired: 2 in, 2 out]
            n145 = property on="Cal Value 2" class="DigNum (strict)"("DisabledEnum"=w221) -> ()  [unwired: 2 in, 2 out]
            n146 = property on="Cal Value 3" class="DigNum (strict)"("DisabledEnum"=w221) -> ()  [unwired: 2 in, 2 out]
            n147 = property on="Cal Value 4" class="DigNum (strict)"("DisabledEnum"=w221) -> ()  [unwired: 2 in, 2 out]
            n148 = property on="Cal Value 5" class="DigNum (strict)"("DisabledEnum"=w221) -> ()  [unwired: 2 in, 2 out]
            n149 = property on="1st Point Cal" class="Bool (strict)"("DisabledEnum"=w221) -> ()  [unwired: 2 in, 2 out]
            n150 = property on="2nd Point Cal" class="Bool (strict)"("DisabledEnum"=w221) -> ()  [unwired: 2 in, 2 out]
            n151 = property on="3rd Point Cal" class="Bool (strict)"("DisabledEnum"=w221) -> ()  [unwired: 2 in, 2 out]
            n152 = property on="4th Point Cal" class="Bool (strict)"("DisabledEnum"=w221) -> ()  [unwired: 2 in, 2 out]
            n153 = Select(t=string[] ["Calibrating 5"], s="5th Point Cal", f=string[] ["Stop Calibrating"]) -> (s? t:f=w222:string[])
          }
          event "Cancel Verify": Value Change {
            n154 = event-data() -> ()  [unwired: 1 in, 1 out]
            n155 = Unbundle By Name(w228) -> ("StreamCtrlActive"=w226:bool, "Desired System.ID"=w227:string)
            n156 = case shown="True" w226 {
              tunnel: w227 -> [_ w230]
              frame False {
              }
              frame True {
                w231 = FALSE
                n157 = Format Into String(format string="ni.var.psp://10.30.189.%s/Streaming Control/StreamCalibrated", w230) -> (resulting string=w237:string, error out=w238:errorcluster)  [unwired: 2 in]
                n158 = shared-variable-open(w237, w238, w231) -> (w232:refnum<k21>, w235:errorcluster)  [unwired: 1 in]
                n159 = shared-variable-write(w232, w235, w231) -> (w233:refnum<k21>, w234:errorcluster)
                n160 = Close Variable Connection(8:w234, 11:w233) -> ()  [unwired: 1 out]
              }
            }
          }
          event "Verify Read": Value Change {
            n161 = event-data() -> ()  [unwired: 1 in, 1 out]
            n162 = case shown="False" "Verify Read" {
              tunnel: [FALSE ("Verify Read") FALSE ("Verify Read")] -> w245
              tunnel: w244 -> [_ _]
              tunnel: w244 -> [w249 w255]
              tunnel: [w249 w254] -> w243
              tunnel: [w247 string[] ["Calc Dev", "Cal Review"]] -> w240
              tunnel: w239 -> [w247 _]
              frame False {
              }
              frame True {
                n163 = local read "Ver Reading"() -> (w250:dbl)
                n164 = local read "Verify Table"() -> (w251:string[][])
                n165 = local read "Row"() -> (w258:i32)
                n166 = Number To Fractional String(number=w250) -> (F-format string=w257:string)  [unwired: 3 in]
                n167 = Replace Array Subset(array=w251, new element=w257, index (row)=w258, index (col)=1 ("disabled index (col)")) -> (w253:string[][])
                n168 = Increment(x=w258) -> (x+1=w262:i32)
                n169 = Bundle(w262, "disabled index (col)"=1) -> (w259:cluster{i32, "disabled index (col)":i32})  [unwired: 1 in]
                n170 = Bundle By Name(cluster=w255, "Verify Table"=w253) -> (w254:T9)
                n171 = property on="Verify Table" class="Tbl (strict)"("Key Focus"=TRUE, "EditPos"=w259, "Value"=w253) -> ()  [unwired: 2 in, 2 out]
              }
            }
            n172 = local write "Verify Read"(w245) -> ()
            n173 = Bundle By Name(cluster=w243, "Init Mean"=TRUE ("initialize")) -> (w242:T9)
          }
          event "Verify Edit": Value Change {
            n174 = event-data() -> ()  [unwired: 1 in, 1 out]
            n175 = case shown="False" "Verify Edit" {
              tunnel: w266 -> [w279 _]
              frame False {
                w280 = T10."Enabled" ("Disabled")
                n176 = Unbundle By Name(w279) -> ("Targets"=w275:T6, "Cal Targets Path"=w277:path, "Cal Unit"=w276:T2)
                n177 = local read "Verify Table"() -> (w278:string[][])
                n178 = Index Array(array=w278, index (col)=0 ("disabled index (col)")) -> (element=w269:string[])  [unwired: 1 in]
                n179 = Fract/Exp String To Number(string=w269) -> (number=w268:dbl[])  [unwired: 3 in, 1 out]
                n180 = Array To Cluster(array=w268) -> (cluster=w267:T14)
                n181 = case shown="\"A\"" w276 {
                  tunnel: w275 -> [w285 w288 w291 w294 w297]
                  tunnel: [w284 w287 w290 w293 w296] -> w274
                  tunnel: w267 -> [w283 w286 w289 w292 w295]
                  frame "V", Default {
                    n182 = Bundle By Name(cluster=w285, "V Targets"=w283) -> (w284:T6)
                  }
                  frame "mA" {
                    n183 = Bundle By Name(cluster=w288, "mA Targets"=w286) -> (w287:T6)
                  }
                  frame "A" {
                    n184 = Bundle By Name(cluster=w291, "A Targets"=w289) -> (w290:T6)
                  }
                  frame "Hz" {
                    n185 = Bundle By Name(cluster=w294, "Hz Targets"=w292) -> (w293:T6)
                  }
                  frame "deg C" {
                    n186 = Bundle By Name(cluster=w297, "TC Targets"=w295) -> (w296:T6)
                  }
                }
                n187 = call <vilib>:"Open Config Data.vi"("configuration file path"=w277) -> ("error out"=w273:errorcluster, "refnum"=w272:T15)  [unwired: 8 in, 1 out]
                n188 = call <userlib>:"Write INI Cluster__ogtk.vi"("error in (no error)"=w273, "INI Fomatted Cluster"=w274, "refnum"=w272) -> ("error out"=w271:errorcluster, "dup refnum"=w270:T15)  [unwired: 7 in]
                n189 = property on="Hide Cal Values" class="Bool"("Visible"=TRUE) -> ()  [unwired: 2 in, 2 out]
                n190 = call <vilib>:"Close Config Data.vi"("error in (no error)"=w271, "refnum"=w270) -> ()  [unwired: 8 in, 2 out]
                n191 = property on="Verify Read" class="Bool (strict)"("DisabledEnum"=w280) -> ()  [unwired: 2 in, 2 out]
                n192 = property on="Auto" class="Bool (strict)"("DisabledEnum"=w280) -> ()  [unwired: 2 in, 2 out]
              }
              frame True {
                w298 = T10."Disabled and Grayed Out" ("Disabled")
                n193 = property on="Verify Read" class="Bool (strict)"("DisabledEnum"=w298) -> ()  [unwired: 2 in, 2 out]
                n194 = property on="Auto" class="Bool (strict)"("DisabledEnum"=w298) -> ()  [unwired: 2 in, 2 out]
                n195 = property on="Hide Cal Values" class="Bool"("Visible"=FALSE) -> ()  [unwired: 2 in, 2 out]
              }
            }
          }
          event "Save Cal": Value Change {
            n196 = event-data() -> ()  [unwired: 1 in, 1 out]
            n197 = property on="Cal Table" class="Tbl (strict)"("DisabledEnum"=T10."Enabled" ("Disabled")) -> ()  [unwired: 2 in, 2 out]
            n198 = property on="Verify Tab" class="TabCtl (strict)"("Visible"=FALSE) -> ()  [unwired: 2 in, 2 out]
          }
          event "Auto": Value Change {
            n199 = event-data() -> ()  [unwired: 1 in, 1 out]
            n200 = case shown="True" "Auto" {
              frame False {
              }
              frame True {
                n201 = local read "Row"() -> (w308:i32)
                n202 = Bundle("Row"=w308, "disabled index (col)"=1) -> (w309:cluster{"Row":i32, "disabled index (col)":i32})  [unwired: 1 in]
                n203 = property on="Verify Table" class="Tbl (strict)"("Key Focus"=TRUE, "EditPos"=w309) -> ()  [unwired: 2 in, 2 out]
              }
            }
            n204 = Bundle By Name(cluster=w306, "Auto"="Auto") -> (w305:T9)
          }
          event "Verify Table": Value Change {
            n205 = event-data() -> ()  [unwired: 1 in, 1 out]
            n206 = Bundle By Name(cluster=w315, "Verify Table"="Verify Table") -> (w314:T9)
          }
          event "Confirm Cal Point": Value Change {
            w320 = T10."Enabled" ("Disabled")
            n207 = event-data() -> ()  [unwired: 1 in, 1 out]
            n208 = local read "Cal Reading"() -> (w324:dbl)
            n209 = Unbundle By Name(w327) -> ("LastCalPt"=w325:i32)
            n210 = flat-sequence {
              tunnel: w325 -> [w331]
              tunnel: w324 -> [w330]
              tunnel: FALSE -> [w329]
              tunnel: "Master Value" -> [w328]
              tunnel: [w347] -> w319
              frame #0 {
                n211 = case shown="0, Default" w331 {
                  tunnel: w330 -> [_ w332 w335 w338 w341 w344]
                  tunnel: w328 -> [_ w334 w337 w340 w343 w346]
                  tunnel: w329 -> [_ w333 w336 w339 w342 w345]
                  frame 0, Default {
                  }
                  frame 1 {
                    n212 = local write "Cal Value 1"(w334) -> ()
                    n213 = local write "1st Point Cal"(w333) -> ()
                    "Reading Value 1" <- w332
                  }
                  frame 2 {
                    n214 = local write "Cal Value 2"(w337) -> ()
                    n215 = local write "2nd Point Cal"(w336) -> ()
                    "Reading Value 2" <- w335
                  }
                  frame 3 {
                    n216 = local write "Cal Value 3"(w340) -> ()
                    n217 = local write "3rd Point Cal"(w339) -> ()
                    "Reading Value 3" <- w338
                  }
                  frame 4 {
                    n218 = local write "Cal Value 4"(w343) -> ()
                    n219 = local write "4th Point Cal"(w342) -> ()
                    "Reading Value 4" <- w341
                  }
                  frame 5 {
                    n220 = local write "Cal Value 5"(w346) -> ()
                    n221 = local write "5th Point Cal"(w345) -> ()
                    "Reading Value 5" <- w344
                  }
                }
              }
              frame #1 {
                n222 = local read "Reading Value 2"() -> (w352:dbl)
                n223 = local read "Reading Value 3"() -> (w353:dbl)
                n224 = local read "Reading Value 4"() -> (w354:dbl)
                n225 = local read "Reading Value 5"() -> (w355:dbl)
                n226 = Not Equal To 0?(x=w352) -> (x != 0?=w351:bool)
                n227 = Not Equal To 0?(x=w353) -> (x != 0?=w350:bool)
                n228 = Not Equal To 0?(x=w354) -> (x != 0?=w349:bool)
                n229 = Not Equal To 0?(x=w355) -> (x != 0?=w348:bool)
                n230 = Compound Arithmetic op=AND(w351, w350, w349, w348) -> (w347:bool)
              }
            }
            n231 = property on="Cal Value 1" class="DigNum (strict)"("DisabledEnum"=w320) -> ()  [unwired: 2 in, 2 out]
            n232 = property on="Cal Value 2" class="DigNum (strict)"("DisabledEnum"=w320) -> ()  [unwired: 2 in, 2 out]
            n233 = property on="Cal Value 3" class="DigNum (strict)"("DisabledEnum"=w320) -> ()  [unwired: 2 in, 2 out]
            n234 = property on="Cal Value 4" class="DigNum (strict)"("DisabledEnum"=w320) -> ()  [unwired: 2 in, 2 out]
            n235 = property on="Cal Value 5" class="DigNum (strict)"("DisabledEnum"=w320) -> ()  [unwired: 2 in, 2 out]
            n236 = property on="1st Point Cal" class="Bool (strict)"("DisabledEnum"=w320) -> ()  [unwired: 2 in, 2 out]
            n237 = property on="2nd Point Cal" class="Bool (strict)"("DisabledEnum"=w320) -> ()  [unwired: 2 in, 2 out]
            n238 = property on="3rd Point Cal" class="Bool (strict)"("DisabledEnum"=w320) -> ()  [unwired: 2 in, 2 out]
            n239 = property on="4th Point Cal" class="Bool (strict)"("DisabledEnum"=w320) -> ()  [unwired: 2 in, 2 out]
            n240 = property on="5th Point Cal" class="Bool (strict)"("DisabledEnum"=w320) -> ()  [unwired: 2 in, 2 out]
            n241 = local write "Cal Tab"(enum32{"Apply", "Cal"}."Apply" ("Cal Tab")) -> ()
            n242 = Select(t=T10."Enabled" ("Disabled"), s=w319, f=T10."Disabled and Grayed Out" ("Disabled")) -> (s? t:f=w316:T10)
            n243 = property on="Apply Cal" class="Bool"("DisabledEnum"=w316) -> ()  [unwired: 2 in, 2 out]
          }
          event "Apply Cal": Value Change {
            n244 = event-data() -> ()  [unwired: 1 in, 6 out]
            n245 = Insert Into Array(array=w359, index=0, new element=string[] ["Calculate Coeffs"]) -> (w358:string[])
          }
          event "Start Verification": Value Change {
            n246 = event-data() -> ()  [unwired: 1 in, 6 out]
            n247 = Unbundle By Name(w363) -> ("StreamCtrlActive"=w361:bool, "Desired System.ID"=w362:string)
            n248 = case shown="True" w361 {
              tunnel: w362 -> [_ w369]
              frame False {
              }
              frame True {
                n249 = Format Into String(format string="ni.var.psp://10.30.189.%s/Streaming Control/StreamCalibrated", w369) -> (resulting string=w377:string, error out=w378:errorcluster)  [unwired: 2 in]
                n250 = shared-variable-open(w377, w378, FALSE) -> (w371:refnum<k21>, w374:errorcluster)  [unwired: 1 in]
                n251 = shared-variable-write(w371, w374, TRUE ("data in")) -> (w372:refnum<k21>, w373:errorcluster)
                n252 = Close Variable Connection(8:w373, 11:w372) -> ()  [unwired: 1 out]
              }
            }
            n253 = property on="Verify Tab" class="TabCtl (strict)"("Visible"="Start Verification") -> ()  [unwired: 2 in, 2 out]
            n254 = Insert Into Array(array=w365, index=0, new element=string[] ["Load Targets", "Calculate Coeffs"]) -> (w364:string[])
          }
          event "Cancel Cal": Value Change {
            w390 = T10."Disabled and Grayed Out" ("Disabled")
            w386 = T10."Enabled" ("Disabled")
            n255 = event-data() -> ()  [unwired: 1 in, 6 out]
            n256 = Unbundle By Name(w382) -> ("Desired System.ID"=w385:string)
            n257 = Format Into String(format string="10.30.189.%s", w385) -> (resulting string=w381:string)  [unwired: 2 in, 1 out]
            n258 = property on="Header" class="Bool"("DisabledEnum"=w386) -> ()  [unwired: 2 in, 2 out]
            n259 = property on="Channel to Cal" class="Enum (strict)"("DisabledEnum"=w386) -> ()  [unwired: 2 in, 2 out]
            n260 = property on="View Spreadsheet" class="Bool"("DisabledEnum"=w386) -> ()  [unwired: 2 in, 2 out]
            n261 = flat-sequence {
              tunnel: w381 -> [w392]
              tunnel: [w392] -> w379
              tunnel: [w395] -> w380
              tunnel: w379 -> [w395]
              frame #0 {
                n262 = local write "RIO Found"(FALSE ("RIO Found")) -> ()
              }
              frame #1 {
                n263 = Wait (ms)(milliseconds to wait=u32 20) -> ()  [unwired: 1 out]
              }
            }
            n264 = property on="Start Cal" class="Bool"("DisabledEnum"=w386) -> ()  [unwired: 2 in, 2 out]
            n265 = disable-structure shown="Disabled" {
              disable-tunnel: w386 -> [w391 _]
              frame Disabled {
                n266 = property on="Start Verification" class="Bool"("DisabledEnum"=w391) -> ()  [unwired: 2 in, 2 out]
              }
              frame Enabled {
              }
            }
            n267 = call "TCP Data Stream PC.vi"("RT IP Address"=w380, "Mode"=TCP_Data_Stream_Mode_(PC)."Close") -> ()  [unwired: 14 in, 4 out]
            n268 = property on="Cal Tab" class="TabCtl (strict)"("Visible"=FALSE) -> ()  [unwired: 2 in, 2 out]
            n269 = property on="Cal Unit" class="Enum (strict)"("DisabledEnum"=T10."Enabled" ("Disabled")) -> ()  [unwired: 2 in, 2 out]
            n270 = property on="Reading Value 1" class="DigNum (strict)"("DisabledEnum"=w390) -> ()  [unwired: 2 in, 2 out]
            n271 = property on="Cal Value 1" class="DigNum (strict)"("DisabledEnum"=w390) -> ()  [unwired: 2 in, 2 out]
            n272 = property on="1st Point Cal" class="Bool (strict)"("DisabledEnum"=w390) -> ()  [unwired: 2 in, 2 out]
            n273 = property on="Reading Value 2" class="DigNum (strict)"("DisabledEnum"=w390) -> ()  [unwired: 2 in, 2 out]
            n274 = property on="Cal Value 2" class="DigNum (strict)"("DisabledEnum"=w390) -> ()  [unwired: 2 in, 2 out]
            n275 = property on="2nd Point Cal" class="Bool (strict)"("DisabledEnum"=w390) -> ()  [unwired: 2 in, 2 out]
            n276 = property on="Reading Value 3" class="DigNum (strict)"("DisabledEnum"=w390) -> ()  [unwired: 2 in, 2 out]
            n277 = property on="Cal Value 3" class="DigNum (strict)"("DisabledEnum"=w390) -> ()  [unwired: 2 in, 2 out]
            n278 = property on="3rd Point Cal" class="Bool (strict)"("DisabledEnum"=w390) -> ()  [unwired: 2 in, 2 out]
            n279 = property on="Reading Value 4" class="DigNum (strict)"("DisabledEnum"=w390) -> ()  [unwired: 2 in, 2 out]
            n280 = property on="Cal Value 4" class="DigNum (strict)"("DisabledEnum"=w390) -> ()  [unwired: 2 in, 2 out]
            n281 = property on="4th Point Cal" class="Bool (strict)"("DisabledEnum"=w390) -> ()  [unwired: 2 in, 2 out]
            n282 = property on="Reading Value 5" class="DigNum (strict)"("DisabledEnum"=w390) -> ()  [unwired: 2 in, 2 out]
            n283 = property on="Cal Value 5" class="DigNum (strict)"("DisabledEnum"=w390) -> ()  [unwired: 2 in, 2 out]
            n284 = property on="5th Point Cal" class="Bool (strict)"("DisabledEnum"=w390) -> ()  [unwired: 2 in, 2 out]
          }
          event "Transfer Cal": Value Change {
            n285 = event-data() -> ()  [unwired: 1 in, 6 out]
            n286 = disable-structure shown="Enabled" {
              disable-tunnel: [string[] ["Distribute Calibration"] w400] -> w397
              disable-tunnel: w396 -> [_ w400]
              frame Disabled {
              }
              frame Enabled {
              }
            }
          }
          event Value Change {
            n287 = event-data() -> ()  [unwired: 1 in, 1 out]
            n288 = Bundle By Name(cluster=w404, "Cal Unit"="Cal Unit") -> (w403:T9)
          }
        }
      }
      frame "Init" {
        w411 = FALSE ("Visible")
        w416 = Units_Type_Def_(DAQ_Rack)."A" ("Cal Unit")
        # "#Change adding in\nnew subVI for RIO"
        n289 = Unbundle By Name(w425) -> ("debug"=w424:bool, "App Dir"=w423:path)
        n290 = Select(t=path "C:/Users/zstreeter/Documents/Projects/Calibration Utility/Source", s=w424, f=w423) -> (s? t:f=w422:path)
        n291 = Build Path(base path=w422, name or relative path="App Config.ini") -> (appended path=w428:path)
        n292 = Build Path(base path=w422, name or relative path="Calibration UIs\\Gas Rack") -> (appended path=w420:path)
        n293 = call "Read App Config.vi"("App Config Path"=w428) -> ("Cal Files Path"=w431:path, "Registered Systems"=w418:T3[])  [unwired: 8 in, 1 out]
        n294 = Build Path(base path=w431, name or relative path="Gas Rack") -> (appended path=w427:path)
        n295 = Build Path(base path=w420, name or relative path="Gas Rack Cal Targets.ini") -> (appended path=w430:path)
        n296 = Create Folder(path (use dialog)=w427) -> (error out=w433:errorcluster)  [unwired: 2 in, 2 out]
        n297 = call <vilib>:"Clear Errors.vi"("error in (no error)"=w433) -> ("error out"=w426:errorcluster)  [unwired: 6 in]
        n298 = for {
          tunnel: [w441] -> w419 mode=indexing
          tunnel: w427 -> [w440]
          tunnel: w426 -> [w439]
          tunnel: w420 -> [w438]
          tunnel: string[] ["Gas Rack Cal Template.xls"] -> [w437] mode=indexing
          n299 = Build Path(base path=w440, name or relative path=w437) -> (appended path=w441:path)
          n300 = Build Path(base path=w438, name or relative path=w437) -> (appended path=w444:path)
          n301 = call <vilib>:"Check if File or Folder Exists.vi"("error in (no error)"=w439, "path"=w441) -> ("file or folder exists?"=w442:bool, "dup path"=w443:path)  [unwired: 7 in, 1 out]
          n302 = case shown="True" w442 {
            tunnel: w443 -> [w446 _]
            tunnel: w444 -> [w445 _]
            frame False {
              n303 = Copy(10:w446, 11:w445) -> ()  [unwired: 3 in, 3 out]
            }
            frame True {
            }
          }
        }
        n304 = Index Array(array=w419) -> (element=w415:path)  [unwired: 1 in]
        n305 = call "Gas Rack Create Cal File Array (RIO).vi"() -> ("Cal Target Array"=w405:string[], "Cal Log OUT"=w406:string[][])  [unwired: 10 in]
        n306 = Bundle By Name(cluster=w425, "Registered Systems"=w418, "Cal Files Base Path"=w427, "Base Path"=w422, "Cal Targets Path"=w430, "Cal Template Path"=w415, "Default Cal Log"=w406, "Cal Target Array"=w405, "Cal Unit"=w416) -> (w410:T9)
        n307 = property on="Cal Tab" class="TabCtl (strict)"("Visible"=w411) -> ()  [unwired: 2 in, 2 out]
        n308 = property on="Verify Tab" class="TabCtl (strict)"("Visible"=w411) -> ()  [unwired: 2 in, 2 out]
        n309 = local write "Tank IP:"("" ("DAQ Rack")) -> ()
        n310 = local write "Cal Table"(string[][] []) -> ()
        n311 = local write "Cal Unit"(w416) -> ()
        n312 = flat-sequence {
          tunnel: w410 -> [w436]
          tunnel: [w436] -> w409
          tunnel: w408 -> [w435]
          frame #0 {
            n313 = Set Occurrence(w435) -> ()
          }
        }
      }
      frame "Unused Items" {
      }
      frame "Init Cal" {
        w451 = FALSE ("Auto")
        w457 = FALSE ("Verify Read")
        w458 = T10."Enabled" ("Disabled")
        w450 = FALSE ("Visible")
        w449 = T10."Disabled and Grayed Out" ("Disabled")
        n314 = Unbundle By Name(w461) -> ("Cal Log Header"=w453:string[])
        n315 = property on="Cal Table" class="Tbl (strict)"("Column Headers[]"=w453) -> ()  [unwired: 2 in, 2 out]
        n316 = property on="Reading Value 1" class="DigNum (strict)"("DisabledEnum"=w449) -> ()  [unwired: 2 in, 2 out]
        n317 = property on="Cal Value 1" class="DigNum (strict)"("DisabledEnum"=w449) -> ()  [unwired: 2 in, 2 out]
        n318 = property on="1st Point Cal" class="Bool (strict)"("DisabledEnum"=w449) -> ()  [unwired: 2 in, 2 out]
        n319 = property on="Reading Value 2" class="DigNum (strict)"("DisabledEnum"=w449) -> ()  [unwired: 2 in, 2 out]
        n320 = property on="Cal Value 2" class="DigNum (strict)"("DisabledEnum"=w449) -> ()  [unwired: 2 in, 2 out]
        n321 = property on="2nd Point Cal" class="Bool (strict)"("DisabledEnum"=w449) -> ()  [unwired: 2 in, 2 out]
        n322 = property on="Reading Value 3" class="DigNum (strict)"("DisabledEnum"=w449) -> ()  [unwired: 2 in, 2 out]
        n323 = property on="Cal Value 3" class="DigNum (strict)"("DisabledEnum"=w449) -> ()  [unwired: 2 in, 2 out]
        n324 = property on="3rd Point Cal" class="Bool (strict)"("DisabledEnum"=w449) -> ()  [unwired: 2 in, 2 out]
        n325 = property on="Reading Value 4" class="DigNum (strict)"("DisabledEnum"=w449) -> ()  [unwired: 2 in, 2 out]
        n326 = property on="Cal Value 4" class="DigNum (strict)"("DisabledEnum"=w449) -> ()  [unwired: 2 in, 2 out]
        n327 = property on="4th Point Cal" class="Bool (strict)"("DisabledEnum"=w449) -> ()  [unwired: 2 in, 2 out]
        n328 = property on="Reading Value 5" class="DigNum (strict)"("DisabledEnum"=w449) -> ()  [unwired: 2 in, 2 out]
        n329 = property on="Cal Value 5" class="DigNum (strict)"("DisabledEnum"=w449) -> ()  [unwired: 2 in, 2 out]
        n330 = property on="5th Point Cal" class="Bool (strict)"("DisabledEnum"=w449) -> ()  [unwired: 2 in, 2 out]
        n331 = property on="Verify Read" class="Bool (strict)"("DisabledEnum"=w458) -> ()  [unwired: 2 in, 2 out]
        n332 = property on="Cal Table" class="Tbl (strict)"("DisabledEnum"=w458) -> ()  [unwired: 2 in, 2 out]
        n333 = property on="Verify Tab" class="TabCtl (strict)"("Visible"=w450) -> ()  [unwired: 2 in, 2 out]
        n334 = property on="Cal Tab" class="TabCtl (strict)"("Visible"=w450) -> ()  [unwired: 2 in, 2 out]
        n335 = property on="Hide Cal Values" class="Bool"("Visible"=TRUE) -> ()  [unwired: 2 in, 2 out]
        n336 = local write "Verify Read"(w457) -> ()
        n337 = local write "Auto"(w457) -> ()
        n338 = local write "Verify Edit"(w457) -> ()
        n339 = Bundle By Name(cluster=w461, "Auto"=w451, "Verification"=w451) -> (w460:T9)
        n340 = Insert Into Array(array=w455, index=0, new element=string[] ["Clear Dev Data", "Update Dev Tables", "Load Template"]) -> (w452:string[])
      }
      frame "Check for RIO" {
        n341 = Unbundle By Name(w469) -> ("Desired System.Serial Number"=w464:string, "StreamCtrlActive"=w462:bool, "Desired System.ID"=w466:string, "Verification"=w467:bool)
        n342 = local read "RIO Found"() -> (w465:bool)
        n343 = local write "Lost Connection"(FALSE ("Lost Connection")) -> ()
        n344 = case shown="False" w465 {
          selector: w465 -> [w475 _]
          tunnel: [string[] [] w483] -> w470
          tunnel: [w475 w482] -> w468
          tunnel: w467 -> [_ w481]
          tunnel: w462 -> [_ w480]
          tunnel: w466 -> [_ w479]
          tunnel: w464 -> [_ w476]
          frame True {
          }
          frame False {
            n345 = call "Find Network Systems.vi"() -> ("Serial Number"=w478:string)  [unwired: 10 in, 1 out]
            n346 = Equal?(x=w478, y=w476) -> (x = y?=w477:bool)
            n347 = case shown="True" w477 {
              selector: w477 -> [w486 w502]
              tunnel: w481 -> [w487 _]
              tunnel: [w488 string[] []] -> w483
              tunnel: [w486 w502] -> w482
              tunnel: w479 -> [w485 _]
              tunnel: w480 -> [w484 _]
              frame True {
                # "Desired system found."
                n348 = case shown="True" w484 {
                  tunnel: w485 -> [_ w489]
                  frame False {
                  }
                  frame True {
                    w490 = FALSE
                    n349 = Format Into String(format string="ni.var.psp://10.30.189.%s/Streaming Control/StreamCalibrated", w489) -> (resulting string=w496:string, error out=w497:errorcluster)  [unwired: 2 in]
                    n350 = shared-variable-open(w496, w497, w490) -> (w491:refnum<k21>, w494:errorcluster)  [unwired: 1 in]
                    n351 = shared-variable-write(w491, w494, w490) -> (w492:refnum<k21>, w493:errorcluster)
                    n352 = Close Variable Connection(8:w493, 11:w492) -> ()  [unwired: 1 out]
                  }
                }
                n353 = case shown="False" w487 {
                  tunnel: [string[] ["Load Targets", "Calculate Coeffs"] w499] -> w488
                  frame True {
                  }
                  frame False {
                    n354 = disable-structure shown="Enabled" {
                      disable-tunnel: [string[] ["Load Targets", "Start Cal"] string[] ["Load Targets"]] -> w499
                      frame Disabled {
                      }
                      frame Enabled {
                      }
                    }
                  }
                }
              }
              frame False {
                # "Couldn't find desired system."
                n355 = property on="Header" class="Bool"("DisabledEnum"=T10."Enabled" ("Disabled")) -> ()  [unwired: 2 in, 2 out]
                n356 = One Button Dialog(message="Couldn't connect to desired DAQ hardware.") -> ()  [unwired: 1 in, 1 out]
              }
            }
          }
        }
        "RIO Found" <- w468
        n357 = Insert Into Array(array=w472, index=0, new element=w470) -> (w471:string[])
      }
      frame "Adjust Channels" {
        n358 = Unbundle By Name(w520) -> ("Cal Unit"=w514:T2)
        n359 = property on="Channel to Cal" class="Enum (strict)"() -> ("NumItems"=w507:u32)  [unwired: 2 in, 2 out]
        n360 = property on="Cal Unit" class="Enum (strict)"() -> ("Strings []"=w517:string[])  [unwired: 2 in, 2 out]
        n361 = for {
          N: w507 -> [_]
          shift-right: [w534] -> w510
          shift-left: i32[] [] ("Disabled Items []") -> [w535]
          i -> [w533]
          n362 = case shown="7" w533 {
            tunnel: w535 -> [w536 w539]
            tunnel: [w536 w537] -> w534
            tunnel: w533 -> [_ w538]
            frame 0..6, Default {
            }
            frame 7 {
              n363 = Build Array (concatenate)(w539, w538) -> (w537:i32[])
            }
          }
        }
        n364 = for {
          tunnel: w517 -> [w528] mode=indexing
          shift-right: [w526] -> w509
          shift-left: i32[] [] ("Disabled Items []") -> [w527]
          i -> [w525]
          n365 = case shown="\"Hz\", \"deg C\", \"mA\"" w528 {
            tunnel: w527 -> [w529 w532]
            tunnel: [w529 w530] -> w526
            tunnel: w525 -> [_ w531]
            frame "A", "V", Default {
            }
            frame "Hz", "deg C", "mA" {
              n366 = Build Array (concatenate)(w532, w531) -> (w530:i32[])
            }
          }
        }
        n367 = Search 1D Array(1D array=w509, element=w514) -> (index of element=w516:i32)  [unwired: 1 in]
        n368 = disable-structure shown="Enabled" {
          disable-tunnel: w510 -> [w523 _]
          disable-tunnel: w509 -> [w522 _]
          disable-tunnel: [w523 w524] -> w506
          disable-tunnel: [w522 w524] -> w508
          frame Disabled {
          }
          frame Enabled {
            w524 = i32[] [] ("Disabled Items []")
          }
        }
        n369 = Greater Or Equal To 0?(x=w516) -> (x >= 0?=w515:bool)
        n370 = case shown="True" w515 {
          tunnel: [w540 w541] -> w513
          tunnel: w514 -> [w540 _]
          tunnel: w509 -> [_ w543]
          frame False {
          }
          frame True {
            n371 = for {
              N: 5 -> [_]
              tunnel: w543 -> [w547]
              tunnel: [w544] -> w541
              i -> [w544]
              stop <- w545 stop-if-true
              n372 = Search 1D Array(1D array=w547, element=w544) -> (index of element=w546:i32)  [unwired: 1 in]
              n373 = Less Than 0?(x=w546) -> (x < 0?=w545:bool)
            }
            n374 = local write "Cal Unit"(w541) -> ()
          }
        }
        n375 = property on="Channel to Cal" class="Enum (strict)"("Disabled Items []"=w506) -> ()  [unwired: 2 in, 2 out]
        n376 = property on="Cal Unit" class="Enum (strict)"("Disabled Items []"=w508) -> ()  [unwired: 2 in, 2 out]
        n377 = Bundle By Name(cluster=w520, "Rack Version"=Rack_Version_Type_Def."RIO", "Cal Unit"=w513) -> (w519:T9)
      }
      frame "Clear Dev Data" {
        n378 = Bundle By Name(cluster=w550, "Verify Table"=string[][] [["", "", "", "", ""], ["", "", "", "", ""], ["", "", "", "", ""], ["", "", "", "", ""], ["", "", "", "", ""], ["", "", "", "", ""], ["", "", "", "", ""], ["", "", "", "", ""], ["", "", "", "", ""], ["", "", "", "", ""]]) -> (w549:T9)
      }
      frame "Update Dev Tables" {
        n379 = Unbundle By Name(w553) -> ("Verify Table"=w552:string[][])
        n380 = local write "Verify Table"(w552) -> ()
      }
      frame "Load Template" {
        n381 = Unbundle By Name(w556) -> ("Cal Template Path"=w561:path)
        n382 = call <vilib>:"Check if File or Folder Exists.vi"("path"=w561) -> ("file or folder exists?"=w560:bool)  [unwired: 8 in, 2 out]
        n383 = case shown="False" w560 {
          tunnel: [string[] [] string[] []] -> w559
          tunnel: w561 -> [w568 w571]
          tunnel: [FALSE ("Visible") FALSE ("Visible")] -> w562
          tunnel: [w565 w573] -> w563
          tunnel: [w565 w573] -> w564
          frame False {
            w565 = T10."Disabled and Grayed Out" ("Disabled")
            n384 = Format Into String(format string="Can't find cal spreadsheet template!\n\nShould have been here:  \"%s\"" ("message"), w568) -> (resulting string=w567:string)  [unwired: 2 in, 1 out]
            n385 = One Button Dialog(message=w567) -> ()  [unwired: 1 in, 1 out]
          }
          frame True {
            w573 = T10."Enabled" ("Disabled")
            n386 = call "Read Write Header.vi"("Cal Template Path"=w571, "Write (F)"=FALSE) -> ("Header Table 1"=w579:string[][], "Header Table 2"=w578:string[][], "Sys Cal Table"=w575:string[][], "Cal Standards Table"=w574:string[][], "Header Comments"=w576:string[][])  [unwired: 13 in]
            n387 = local write "Header Table 1"(w579) -> ()
            n388 = local write "Header Table 2"(w578) -> ()
            n389 = local write "Sys Cal Table"(w575) -> ()
            n390 = local write "Cal Standards Table"(w574) -> ()
            n391 = local write "Header Comments"(w576) -> ()
          }
        }
        n392 = property on="Load Indicator Tab" class="TabCtl (strict)"("Visible"=w562) -> ()  [unwired: 2 in, 2 out]
        n393 = property on="Header OK" class="Bool"("DisabledEnum"=w563) -> ()  [unwired: 2 in, 2 out]
        n394 = property on="Header Cancel" class="Bool"("DisabledEnum"=w564) -> ()  [unwired: 2 in, 2 out]
        n395 = Insert Into Array(array=w558, index=0, new element=w559) -> (w557:string[])
      }
      frame "Create Spreadsheet" {
        n396 = Unbundle By Name(w592) -> ("Rack Version"=w587:T5, "DAQ Rack"=w584:string, "Cal Files Base Path"=w594:path)
        n397 = Format Into String(format string="%s.xls", w584) -> (resulting string=w583:string)  [unwired: 2 in, 1 out]
        n398 = case shown="\"RIO\"" w587 {
          tunnel: ["DAQ Rack Cal Template.xls" ("name or relative path") "DAQ Cart Cal Template.xls" ("name or relative path") "Gas Rack Cal Template.xls" ("name or relative path")] -> w582
          frame Default {
          }
          frame "Cart" {
          }
          frame "RIO" {
          }
        }
        n399 = Build Path(base path=w594, name or relative path=w583) -> (appended path=w581:path)
        n400 = Empty String/Path?(string/path=w584) -> (empty?=w586:bool)
        n401 = Not A Number/Path/Refnum?(number/path/refnum=w581) -> (NaN/Path/Refnum?=w596:bool)
        n402 = Or(x=w596, y=w586) -> (x .or. y?=w597:bool)
        n403 = Build Path(base path=w594, name or relative path=w582) -> (appended path=w595:path)
        n404 = case shown="False" w597 {
          tunnel: [string[] ["Save Header"] string[] []] -> w593
          tunnel: w581 -> [w602 _]
          tunnel: w595 -> [w603 _]
          frame False {
            n405 = call <vilib>:"Check if File or Folder Exists.vi"("path"=w602) -> ("file or folder exists?"=w601:bool)  [unwired: 8 in, 2 out]
            n406 = case shown="False" w601 {
              tunnel: w602 -> [w607 _]
              tunnel: w603 -> [w606 _]
              frame False {
                n407 = Copy(9:TRUE ("overwrite (F)"), 10:w607, 11:w606) -> ()  [unwired: 2 in, 3 out]
              }
              frame True {
              }
            }
          }
          frame True {
            w608 = T10."Enabled" ("Disabled")
            n408 = property on="Load Indicator Tab" class="TabCtl (strict)"("Visible"=FALSE) -> ()  [unwired: 2 in, 2 out]
            n409 = property on="Header OK" class="Bool"("DisabledEnum"=w608) -> ()  [unwired: 2 in, 2 out]
            n410 = property on="Header Cancel" class="Bool"("DisabledEnum"=w608) -> ()  [unwired: 2 in, 2 out]
            n411 = One Button Dialog(message="\"Manufacturer Serial #\" is blank or contains invalid characters.") -> ()  [unwired: 1 in, 1 out]
          }
        }
        n412 = Bundle By Name(cluster=w592, "Cal Spreadsheet Path"=w581) -> (w591:T9)
        n413 = Insert Into Array(array=w589, index=0, new element=w593) -> (w590:string[])
      }
      frame "Save Header" {
        n414 = Unbundle By Name(w620) -> ("Cal Spreadsheet Path"=w623:path, "Cal Template Path"=w624:path)
        n415 = Build Array(w623, w624) -> (w625:path[])
        n416 = for {
          tunnel: "Header Table 2" -> [w633]
          tunnel: "Sys Cal Table" -> [w632]
          tunnel: "Cal Standards Table" -> [w631]
          tunnel: "Header Comments" -> [w630]
          tunnel: [w629] -> w622
          tunnel: "Header Table 1" -> [w627]
          tunnel: w625 -> [w626] mode=indexing
          n417 = call "Read Write Header.vi"("Header Table 1 IN"=w627, "Header Table 2 IN"=w633, "Sys Cal Table IN"=w632, "Cal Standards Table IN"=w631, "Header Comments IN"=w630, "Cal Template Path"=w626, "Write (F)"=TRUE) -> ("Header Table 1"=w629:string[][])  [unwired: 8 in, 4 out]
        }
        n418 = flat-sequence {
          tunnel: w622 -> [_]
          frame #0 {
            w634 = T10."Enabled" ("Disabled")
            w636 = FALSE ("Visible")
            n419 = disable-structure shown="Disabled" {
              disable-tunnel: w634 -> [w637 _]
              frame Disabled {
                n420 = property on="Start Verification" class="Bool"("DisabledEnum"=w637) -> ()  [unwired: 2 in, 2 out]
              }
              frame Enabled {
              }
            }
            n421 = property on="View Spreadsheet" class="Bool"("DisabledEnum"=w634) -> ()  [unwired: 2 in, 2 out]
            n422 = property on="Main Tab" class="TabCtl (strict)"("DisabledEnum"=w634) -> ()  [unwired: 2 in, 2 out]
            n423 = property on="Tank IP:" class="Str"("DisabledEnum"=w634) -> ()  [unwired: 2 in, 2 out]
            n424 = property on="Channel to Cal" class="Enum (strict)"("DisabledEnum"=w634) -> ()  [unwired: 2 in, 2 out]
            n425 = property on="Start Cal" class="Bool"("DisabledEnum"=w634) -> ()  [unwired: 2 in, 2 out]
            n426 = property on="Cal Unit" class="Enum (strict)"("DisabledEnum"=T10."Enabled" ("Disabled")) -> ()  [unwired: 2 in, 2 out]
            n427 = property on="Load Indicator Tab" class="TabCtl (strict)"("Visible"=w636) -> ()  [unwired: 2 in, 2 out]
            n428 = property on="Header Tab" class="TabCtl (strict)"("Visible"=w636) -> ()  [unwired: 2 in, 2 out]
          }
        }
        n429 = Insert Into Array(array=w618, index=0, new element=string[] []) -> (w619:string[])
      }
      frame "Create Cal File" {
        n430 = Unbundle By Name(w641) -> ("Cal Files Base Path"=w643:path, "Cal Log Header"=w646:string[], "Default Cal Log"=w645:string[][])
        n431 = local read "Tank IP:"() -> (w638:string)
        n432 = Build Array (concatenate)(w646, w645) -> (w644:string[][])
        n433 = case shown="Default" w638 {
          tunnel: w644 -> [w655 _]
          tunnel: w643 -> [w654 _]
          tunnel: w638 -> [w652 _]
          tunnel: [w653 path "" ("dup path")] -> w639
          frame Default {
            n434 = Format Into String(format string="%s.cal", w652) -> (resulting string=w650:string)  [unwired: 2 in, 1 out]
            n435 = Build Path(base path=w654, name or relative path=w650) -> (appended path=w658:path)
            n436 = call <vilib>:"Check if File or Folder Exists.vi"("path"=w658) -> ("file or folder exists?"=w657:bool, "dup path"=w656:path)  [unwired: 8 in, 1 out]
            n437 = case shown="False" w657 {
              tunnel: w656 -> [w662 w663]
              tunnel: w655 -> [w661 _]
              tunnel: [w659 w663] -> w653
              frame False {
                n438 = call-poly <vilib>:"Write To Spreadsheet File.vi"("delimiter (\\t)"="," ("delimiter (\\t)"), "2D data"=w661, "file path (dialog if empty)"=w662) -> ("new file path (Not A Path if cancelled)"=w659:path)  [unwired: 5 in]
              }
              frame True {
              }
            }
          }
          frame "" {
          }
        }
        n439 = Bundle By Name(cluster=w641, "Cal File Path"=w639) -> (w640:T9)
        n440 = Insert Into Array(array=w647, index=0, new element=string[] ["Load Cal File"]) -> (w648:string[])
      }
      frame "Load Cal File" {
        n441 = Unbundle By Name(w669) -> ("Default Cal Log"=w665:string[][], "Cal File Path"=w666:path)
        n442 = Empty String/Path?(string/path=w666) -> (empty?=w667:bool)
        n443 = case shown="False" w667 {
          tunnel: w666 -> [w676 _]
          tunnel: [w680 w717] -> w673
          tunnel: [w678 string[] []] -> w670
          tunnel: w669 -> [w677 w717]
          tunnel: w665 -> [w674 _]
          frame False {
            n444 = call <vilib>:"Check if File or Folder Exists.vi"("path"=w676) -> ("file or folder exists?"=w679:bool, "dup path"=w675:path)  [unwired: 8 in, 1 out]
            n445 = case shown="True" w679 {
              tunnel: w675 -> [_ w711]
              tunnel: w677 -> [w681 w708]
              tunnel: [w681 w707] -> w680
              tunnel: [string[] ["Create Cal File"] string[] []] -> w678
              tunnel: w674 -> [_ w704]
              frame False {
              }
              frame True {
                w703 = 0 ("index (row)")
                n446 = call-poly <vilib>:"Read From Spreadsheet File.vi"("delimiter (\\t)"="," ("delimiter (\\t)"), "file path (dialog if empty)"=w711) -> ("all rows"=w710:string[][])  [unwired: 5 in, 4 out]
                n447 = Delete From Array(array=w710, index (row)=0) -> (array with subset deleted=w699:string[][])  [unwired: 2 in, 1 out]
                n448 = Index Array(array=w699, index (col)=0 ("disabled index (col)")) -> (element=w701:string[])  [unwired: 1 in]
                n449 = Search 1D Array(1D array=w701, element="") -> (index of element=w697:i32)  [unwired: 1 in]
                n450 = Delete From Array(array=w699, index (row)=w697) -> (array with subset deleted=w698:string[][])  [unwired: 2 in, 1 out]
                n451 = Replace Array Subset(array=w704, new element=w698, index (row)=w703, index (col)=w703) -> (w691:string[][])
                n452 = Index Array(array=w691, index (col)=1 ("disabled index (col)")) -> (element=w684:string[])  [unwired: 1 in]
                n453 = for {
                  tunnel: w684 -> [w713] mode=indexing
                  tunnel: [w712] -> w683 mode=indexing
                  n454 = case shown="\"V\", Default" w713 {
                    tunnel: ["V" "A"] -> w712
                    frame "V", Default {
                    }
                    frame "A" {
                    }
                  }
                }
                n455 = Array To Spreadsheet String(array=w683, 3:"%s" ("format string")) -> (spreadsheet string=w695:string)  [unwired: 1 in]
                n456 = Search and Replace String(replace all?=TRUE ("replace all? (F)"), input string=w695, search string="degC", replace string="deg C" ("search string")) -> (result string=w688:string)  [unwired: 4 in, 3 out]
                n457 = Spreadsheet String To Array(format string="%s", spreadsheet string=w688, array type (2D Dbl)=w683) -> (array=w687:string[])  [unwired: 1 in]
                n458 = Replace Array Subset(array=w691, new element=w687, index (col)=1 ("disabled index (col)")) -> (w690:string[][])  [unwired: 1 in]
                n459 = Bundle By Name(cluster=w708, "Cal Log"=w690) -> (w707:T9)
                n460 = property on="Cal Table" class="Tbl (strict)"("Value"=w690) -> ()  [unwired: 2 in, 2 out]
              }
            }
          }
          frame True {
          }
        }
        n461 = Insert Into Array(array=w671, index=0, new element=w670) -> (w672:string[])
      }
      frame "Load Targets" {
        w774 = 0 ("length")
        # "#Change In \"A\" selection added selection of \"RIO\" that links 25A Targets and Setpoints"
        n462 = Unbundle By Name(w777) -> ("Cal Log"=w742:string[][], "Cal Targets Path"=w784:path, "Targets"=w779:T6, "Cal Target Array"=w764:string[], "Verify Table"=w731:string[][], "Channel to Cal"=w753:T1)
        n463 = property on="Cancel Verify" class="Bool"("DisabledEnum"=T10."Enabled" ("Disabled")) -> ()  [unwired: 2 in, 2 out]
        n464 = property on="Cal Table" class="Tbl (strict)"("Active Cell"=T12 {"Row"=-2, "Column"=-2} ("Active Cell:Active Cell"), "Cell BG Color"=u32 16448250) -> ()  [unwired: 2 in, 2 out]
        n465 = Index Array(array=w742, index (row)=w753) -> (element=w763:string[])  [unwired: 1 in]
        n466 = call <vilib>:"Open Config Data.vi"("configuration file path"=w784) -> ("error out"=w782:errorcluster, "refnum"=w783:T15)  [unwired: 8 in, 1 out]
        n467 = Array Subset "Calibration"(array=w763, index=2, length=10) -> (w726:string[])
        n468 = Array Subset "Verification"(array=w763, index=18, length=20) -> (w733:string[])
        n469 = property on="Apply Cal" class="Bool"("DisabledEnum"=T10."Disabled and Grayed Out" ("Disabled")) -> ()  [unwired: 2 in, 2 out]
        n470 = call <userlib>:"Read INI Cluster__ogtk.vi"("error in (no error)"=w782, "INI Fomatted Cluster Type"=w779, "refnum"=w783) -> ("error out"=w780:errorcluster, "INI Fomatted Cluster"=w778:variant, "dup refnum"=w781:T15)  [unwired: 4 in, 2 out]
        n471 = Index Array(array=w733, index #1=1 ("index"), index #2=3 ("index"), index #3=5 ("index"), index #4=7 ("index"), index #5=9 ("index")) -> (element #1=w752:string, element #2=w749:string, element #3=w751:string, element #4=w748:string, element #5=w750:string)
        n472 = call <vilib>:"Close Config Data.vi"("error in (no error)"=w780, "refnum"=w781) -> ()  [unwired: 8 in, 2 out]
        n473 = Fract/Exp String To Number(string=w726) -> (number=w736:dbl[])  [unwired: 3 in, 1 out]
        n474 = Empty Array?(array=w726) -> ()  [unwired: 1 out]
        n475 = Empty String/Path?(string/path=w752) -> (empty?=w745:bool)
        n476 = Empty String/Path?(string/path=w751) -> (empty?=w744:bool)
        n477 = Empty String/Path?(string/path=w750) -> (empty?=w743:bool)
        n478 = Variant To Data(type=w779, Variant=w778) -> (data=w767:T6)  [unwired: 1 in, 1 out]
        n479 = Index Array(array=w764, index=w753) -> (element=w768:string)
        n480 = Empty String/Path?(string/path=w749) -> (empty?=w747:bool)
        n481 = Empty String/Path?(string/path=w748) -> (empty?=w746:bool)
        n482 = Compound Arithmetic op=AND(w745, w747, w744, w746, w743) -> (w727:bool)
        n483 = case shown="\"DegC\"" w768 {
          tunnel: w767 -> [w832 w835 w838 w841 w844 w847]
          tunnel: [w830 w833 w836 w839 w842 w845] -> w765
          tunnel: [w831 w834 w837 w840 w843 w846] -> w766
          frame "V", Default {
            n484 = Unbundle By Name(w832) -> ("V Targets"=w831:T7, "V Setpoints"=w830:T8)
          }
          frame "A" {
            n485 = Unbundle By Name(w835) -> ("A Targets"=w834:T7, "A Setpoints"=w833:T8)
          }
          frame "DegC" {
            n486 = Unbundle By Name(w838) -> ("DegC Targets"=w837:T7, "DegC Setpoints"=w836:T8)
          }
          frame "kPa" {
            n487 = Unbundle By Name(w841) -> ("kPa Targets"=w840:T7, "kPa Setpoints"=w839:T8)
          }
          frame "LpH" {
            n488 = Unbundle By Name(w844) -> ("LpH Targets"=w843:T7, "LpH Setpoints"=w842:T8)
          }
          frame "CT" {
            n489 = Unbundle By Name(w847) -> ("CT Targets"=w846:T7, "CT Setpoints"=w845:T8)
          }
        }
        n490 = case shown="True" w727 {
          tunnel: w733 -> [_ w805]
          tunnel: w731 -> [w797 w804]
          tunnel: [w797 w798] -> w730
          frame True {
          }
          frame False {
            n491 = for {
              tunnel: w805 -> [w811] mode=indexing
              tunnel: [w811] -> w800 mode=indexing if=w807
              tunnel: [w811] -> w799 mode=indexing if=w806
              i -> [w810]
              n492 = Quotient & Remainder(x=w810, y=2) -> (x-y*floor(x/y)=w808:i32)  [unwired: 1 out]
              n493 = Equal To 0?(x=w808) -> (x = 0?=w807:bool)
              n494 = Not(x=w807) -> (.not. x?=w806:bool)
            }
            n495 = Replace Array Subset(array=w804, new element=w800, index (col)=0 ("disabled index (col)")) -> (w803:string[][])  [unwired: 1 in]
            n496 = Replace Array Subset(array=w803, new element=w799, index (col)=1 ("disabled index (col)")) -> (w798:string[][])  [unwired: 1 in]
          }
        }
        n497 = case shown="False" w727 {
          tunnel: w729 -> [w794 w796]
          tunnel: [w793 w796] -> w728
          frame False {
            n498 = Insert Into Array(array=w794, index=0, new element=string[] ["Calc Dev"]) -> (w793:string[])
          }
          frame True {
          }
        }
        n499 = for {
          tunnel: w726 -> [w791] mode=indexing
          tunnel: [w790] -> w725 mode=indexing
          n500 = Empty String/Path?(string/path=w791) -> (empty?=w790:bool)
        }
        n501 = Cluster To Array(cluster=w766) -> (array=w775:dbl[])
        n502 = Cluster To Array(cluster=w765) -> (array=w732:dbl[])
        n503 = And Array Elements(Boolean array=w725) -> (logical AND=w724:bool)
        n504 = Delete From Array(array=w775, length=w774, index=w774) -> (deleted portion=w770:dbl[], array with subset deleted=w773:dbl[])
        n505 = call-poly <userlib>:"Remove Duplicates from 1D Array__ogtk.vi"("Input Array"=w773) -> ("Output Array"=w772:dbl[])  [unwired: 1 out]
        n506 = Build Array (concatenate)(w770, w772) -> (w771:dbl[])
        n507 = Number To Fractional String(number=w771, precision (6)=i16 3) -> (F-format string=w776:string[])  [unwired: 2 in]
        n508 = case shown="False" w724 {
          tunnel: w732 -> [_ w829]
          tunnel: [w817 w828] -> w741
          tunnel: [w821 w827] -> w740
          tunnel: [w820 w826] -> w739
          tunnel: [w819 w825] -> w738
          tunnel: [w818 w824] -> w737
          tunnel: w736 -> [w822 _]
          tunnel: [w816 w823] -> w723
          tunnel: [w815 w823] -> w722
          tunnel: [w814 w823] -> w721
          tunnel: [w813 w823] -> w720
          tunnel: [w812 w823] -> w719
          frame False {
            n509 = Index Array(array=w822) -> (element #1=w816:dbl, element #2=w821:dbl, element #3=w815:dbl, element #4=w820:dbl, element #5=w814:dbl, element #6=w819:dbl, element #7=w813:dbl, element #8=w818:dbl, element #9=w812:dbl, element #10=w817:dbl)  [unwired: 10 in]
          }
          frame True {
            w823 = 0.0 ("Label")
            n510 = Index Array(array=w829) -> (element #1=w827:dbl, element #2=w826:dbl, element #3=w825:dbl, element #4=w824:dbl, element #5=w828:dbl)  [unwired: 5 in]
          }
        }
        n511 = Replace Array Subset(array=w731, new element=w776, index (col)=0 ("disabled index (col)")) -> (w735:string[][])  [unwired: 1 in]
        n512 = Select(t=w735, s=w727, f=w730) -> (s? t:f=w734:string[][])
        n513 = local write "Reading Value 1"(w723) -> ()
        n514 = local write "Reading Value 2"(w722) -> ()
        n515 = local write "Reading Value 3"(w721) -> ()
        n516 = local write "Reading Value 4"(w720) -> ()
        n517 = local write "Reading Value 5"(w719) -> ()
        n518 = local write "Cal Value 1"(w740) -> ()
        n519 = local write "Cal Value 2"(w739) -> ()
        n520 = local write "Cal Value 3"(w738) -> ()
        n521 = local write "Cal Value 4"(w737) -> ()
        n522 = local write "Cal Value 5"(w741) -> ()
        n523 = Bundle By Name(cluster=w777, "Targets"=w767, "Verify Table"=w734) -> (w786:T9)
        n524 = property on="Verify Table" class="Tbl (strict)"("Value"=w734) -> ()  [unwired: 2 in, 2 out]
      }
      frame "Start Cal" {
        w848 = T10."Disabled and Grayed Out" ("Disabled")
        w851 = T10."Enabled" ("Disabled")
        n525 = property on="Header" class="Bool"("DisabledEnum"=w848) -> ()  [unwired: 2 in, 2 out]
        n526 = property on="Channel to Cal" class="Enum (strict)"("DisabledEnum"=w848) -> ()  [unwired: 2 in, 2 out]
        n527 = property on="View Spreadsheet" class="Bool"("DisabledEnum"=w848) -> ()  [unwired: 2 in, 2 out]
        n528 = property on="Cal Tab" class="TabCtl (strict)"("Visible"=TRUE) -> ()  [unwired: 2 in, 2 out]
        n529 = property on="Start Cal" class="Bool"("DisabledEnum"=w848) -> ()  [unwired: 2 in, 2 out]
        n530 = disable-structure shown="Disabled" {
          disable-tunnel: w848 -> [w853 _]
          frame Disabled {
            n531 = property on="Cal Unit" class="Enum (strict)"("DisabledEnum"=w853) -> ()  [unwired: 2 in, 2 out]
          }
          frame Enabled {
          }
        }
        n532 = property on="Start Verification" class="Bool"("DisabledEnum"=w848) -> ()  [unwired: 2 in, 2 out]
        n533 = property on="Reading Value 1" class="DigNum (strict)"("DisabledEnum"=w851) -> ()  [unwired: 2 in, 2 out]
        n534 = property on="Cal Value 1" class="DigNum (strict)"("DisabledEnum"=w851) -> ()  [unwired: 2 in, 2 out]
        n535 = property on="1st Point Cal" class="Bool (strict)"("DisabledEnum"=w851) -> ()  [unwired: 2 in, 2 out]
        n536 = property on="Reading Value 2" class="DigNum (strict)"("DisabledEnum"=w851) -> ()  [unwired: 2 in, 2 out]
        n537 = property on="Cal Value 2" class="DigNum (strict)"("DisabledEnum"=w851) -> ()  [unwired: 2 in, 2 out]
        n538 = property on="2nd Point Cal" class="Bool (strict)"("DisabledEnum"=w851) -> ()  [unwired: 2 in, 2 out]
        n539 = property on="Reading Value 3" class="DigNum (strict)"("DisabledEnum"=w851) -> ()  [unwired: 2 in, 2 out]
        n540 = property on="Cal Value 3" class="DigNum (strict)"("DisabledEnum"=w851) -> ()  [unwired: 2 in, 2 out]
        n541 = property on="3rd Point Cal" class="Bool (strict)"("DisabledEnum"=w851) -> ()  [unwired: 2 in, 2 out]
        n542 = property on="Reading Value 4" class="DigNum (strict)"("DisabledEnum"=w851) -> ()  [unwired: 2 in, 2 out]
        n543 = property on="Cal Value 4" class="DigNum (strict)"("DisabledEnum"=w851) -> ()  [unwired: 2 in, 2 out]
        n544 = property on="4th Point Cal" class="Bool (strict)"("DisabledEnum"=w851) -> ()  [unwired: 2 in, 2 out]
        n545 = property on="Reading Value 5" class="DigNum (strict)"("DisabledEnum"=w851) -> ()  [unwired: 2 in, 2 out]
        n546 = property on="Cal Value 5" class="DigNum (strict)"("DisabledEnum"=w851) -> ()  [unwired: 2 in, 2 out]
        n547 = property on="5th Point Cal" class="Bool (strict)"("DisabledEnum"=w851) -> ()  [unwired: 2 in, 2 out]
      }
      frame "Calibrating 1".."Calibrating 6" {
        # "When it said \"Calibrating 1\"..\"Calibrating 5\" it was not accepting Calibrating 5"
        n548 = case shown="\"Calibrating 4\"" w859 {
          tunnel: [0.0 w865 w867 w869 w871 w873] -> w858
          tunnel: [1 1 2 3 4 5] -> w854
          frame Default {
          }
          frame "Calibrating 1" {
            n549 = local read "Cal Value 1"() -> (w865:dbl)
          }
          frame "Calibrating 2" {
            n550 = local read "Cal Value 2"() -> (w867:dbl)
          }
          frame "Calibrating 3" {
            n551 = local read "Cal Value 3"() -> (w869:dbl)
          }
          frame "Calibrating 4" {
            n552 = local read "Cal Value 4"() -> (w871:dbl)
          }
          frame "Calibrating 5" {
            n553 = local read "Cal Value 5"() -> (w873:dbl)
          }
        }
        n554 = property on="Cal Tab" class="TabCtl (strict)"("Visible"=TRUE) -> ()  [unwired: 2 in, 2 out]
        n555 = local write "Cal Tab"(enum32{"Apply", "Cal"}."Cal" ("Cal Tab")) -> ()
        n556 = local write "Master Value"(w858) -> ()
        n557 = Bundle By Name(cluster=w856, "LastCalPt"=w854) -> (w855:T9)
      }
      frame "Stop Calibrating" {
        n558 = local write "Cal Tab"(enum32{"Apply", "Cal"}."Apply" ("Cal Tab")) -> ()
      }
      frame "Calculate Coeffs" {
        w878 = T10."Enabled" ("Disabled")
        # "Used to enable and start the verification from here"
        n559 = Unbundle By Name(w885) -> ("Channel to Cal"=w881:T1, "Cal Unit"=w884:T2, "Verification"=w883:bool, "Cal Log"=w882:string[][])
        n560 = case shown="False" w883 {
          tunnel: [w899 w926] -> w890
          tunnel: [w898 w925] -> w889
          tunnel: [w897 w924] -> w888
          tunnel: w884 -> [w896 w923]
          tunnel: w882 -> [_ w927]
          tunnel: w881 -> [_ w928]
          tunnel: [w895 w922] -> w880
          tunnel: [w894 w921] -> w879
          frame False {
            n561 = case shown="\"V\", \"Hz\", Default" w896 {
              tunnel: [w916 w919] -> w899
              tunnel: [w915 1.0] -> w898
              tunnel: [w914 w919] -> w897
              tunnel: [w909 w919] -> w895
              tunnel: [w908 w919] -> w894
              frame "V", "Hz", Default {
                n562 = local read "Reading Value 1"() -> (w907:dbl)
                n563 = local read "Reading Value 2"() -> (w906:dbl)
                n564 = local read "Reading Value 3"() -> (w905:dbl)
                n565 = local read "Reading Value 4"() -> (w903:dbl)
                n566 = local read "Reading Value 5"() -> (w902:dbl)
                n567 = Build Array("Cal Value 1", "Cal Value 2", "Cal Value 3", "Cal Value 4", "Cal Value 5") -> (w913:dbl[])
                n568 = Build Array(w907, w906, w905, w903, w902) -> (w912:dbl[])
                n569 = call <vilib>:"General Polynomial Fit Coefficients.vi"("Y"=w913, "polynomial order"=4, "X"=w912) -> ("Polynomial Coefficients"=w911:dbl[])  [unwired: 11 in, 1 out]
                n570 = Index Array(array=w911) -> (element #1=w916:dbl, element #2=w915:dbl, element #3=w914:dbl, element #4=w909:dbl, element #5=w908:dbl)  [unwired: 5 in]
              }
              frame "deg C" {
                w919 = 0.0
              }
            }
          }
          frame True {
            n571 = case shown="Default" w923 {
              selector: w923 -> [w931 _]
              tunnel: w928 -> [w947 _]
              tunnel: w927 -> [w939 _]
              tunnel: [w934 w953] -> w926
              tunnel: [w933 1.0 ("Label")] -> w925
              tunnel: [w932 w953] -> w924
              tunnel: [w930 w953] -> w922
              tunnel: [w929 w953] -> w921
              frame Default {
                n572 = Format Into String(w947) -> (resulting string=w944:string)  [unwired: 3 in, 1 out]
                n573 = Format Into String(w931) -> (resulting string=w940:string)  [unwired: 3 in, 1 out]
                n574 = Index Array(array=w939, index (col) #1=0 ("disabled index (col)"), index (col) #2=1 ("index (col)")) -> (element #1=w945:string[], element #2=w941:string[])  [unwired: 2 in]
                n575 = call-poly <userlib>:"Search Array__ogtk.vi"("Array"=w945, "Element Data"=w944) -> ("Indices of Elements"=w942:i32[])  [unwired: 7 in]
                n576 = for {
                  tunnel: w942 -> [w948] mode=indexing
                  tunnel: w941 -> [w952]
                  tunnel: w940 -> [w950]
                  tunnel: [w948] -> w938
                  stop <- w949 stop-if-true
                  n577 = Index Array(array=w952, index=w948) -> (element=w951:string)
                  n578 = Equal?(x=w950, y=w951) -> (x = y?=w949:bool)
                }
                n579 = Index Array(array=w939, index (row)=w938) -> (element=w937:string[])  [unwired: 1 in]
                n580 = Fract/Exp String To Number(string=w937) -> (number=w936:dbl[])  [unwired: 3 in, 1 out]
                n581 = Index Array(array=w936, index #1=12 ("index")) -> (element #1=w934:dbl, element #2=w933:dbl, element #3=w932:dbl, element #4=w930:dbl, element #5=w929:dbl)  [unwired: 4 in]
              }
              frame "deg C" {
                w953 = 0.0 ("Label")
              }
            }
          }
        }
        "a0" <- w890
        "a2" <- w888
        "a1" <- w889
        "a4" <- w879
        "a3" <- w880
        n582 = property on="Cal Table" class="Tbl (strict)"("DisabledEnum"=T10."Disabled and Grayed Out" ("Disabled")) -> ()  [unwired: 2 in, 2 out]
        n583 = property on="Save Cal" class="Bool"("DisabledEnum"=T10."Enabled" ("Disabled")) -> ()  [unwired: 2 in, 2 out]
        n584 = Insert Into Array(array=w891, index=0, new element=string[] ["Save Calibration"]) -> (w892:string[])
        n585 = property on="a0" class="DigNum (strict)"("DisabledEnum"=w878) -> ()  [unwired: 2 in, 2 out]
        n586 = property on="a1" class="DigNum (strict)"("DisabledEnum"=w878) -> ()  [unwired: 2 in, 2 out]
        n587 = property on="a2" class="DigNum (strict)"("DisabledEnum"=w878) -> ()  [unwired: 2 in, 2 out]
        n588 = property on="a3" class="DigNum (strict)"("DisabledEnum"=w878) -> ()  [unwired: 2 in, 2 out]
        n589 = property on="a4" class="DigNum (strict)"("DisabledEnum"=w878) -> ()  [unwired: 2 in, 2 out]
      }
      frame "Cal Review Prep" {
        w960 = T10."Disabled and Grayed Out" ("Disabled")
        n590 = Unbundle By Name(w961) -> ("Desired System.ID"=w962:string)
        n591 = Format Into String(format string="ni.var.psp://10.30.189.%s/Streaming Control/StreamCalibrated", w962) -> (resulting string=w970:string, error out=w971:errorcluster)  [unwired: 2 in]
        n592 = property on="Cal Tab" class="TabCtl (strict)"("Visible"=FALSE) -> ()  [unwired: 2 in, 2 out]
        n593 = property on="Verify Tab" class="TabCtl (strict)"("Visible"=TRUE) -> (error out=w957:errorcluster)  [unwired: 2 in, 1 out]
        n594 = shared-variable-open(w970, w971, FALSE) -> (w964:refnum<k21>, w967:errorcluster)  [unwired: 1 in]
        n595 = shared-variable-write(w964, w967, TRUE ("data in")) -> (w965:refnum<k21>, w966:errorcluster)
        n596 = property on="Verify Table" class="Tbl (strict)"(error in=w957, "Key Focus"=TRUE, "EditPos"=T12 {"Row"=0, "Column"=1} ("Active Cell:Active Cell")) -> ()  [unwired: 1 in, 2 out]
        n597 = Close Variable Connection(8:w966, 11:w965) -> ()  [unwired: 1 out]
        n598 = Insert Into Array(array=w975, index=0, new element=string[] ["Cal Review"]) -> (w974:string[])
        n599 = property on="Reading Value 1" class="DigNum (strict)"("DisabledEnum"=w960) -> ()  [unwired: 2 in, 2 out]
        n600 = property on="Cal Value 1" class="DigNum (strict)"("DisabledEnum"=w960) -> ()  [unwired: 2 in, 2 out]
        n601 = property on="1st Point Cal" class="Bool (strict)"("DisabledEnum"=w960) -> ()  [unwired: 2 in, 2 out]
        n602 = property on="Reading Value 2" class="DigNum (strict)"("DisabledEnum"=w960) -> ()  [unwired: 2 in, 2 out]
        n603 = property on="Cal Value 2" class="DigNum (strict)"("DisabledEnum"=w960) -> ()  [unwired: 2 in, 2 out]
        n604 = property on="2nd Point Cal" class="Bool (strict)"("DisabledEnum"=w960) -> ()  [unwired: 2 in, 2 out]
        n605 = property on="Reading Value 3" class="DigNum (strict)"("DisabledEnum"=w960) -> ()  [unwired: 2 in, 2 out]
        n606 = property on="Cal Value 3" class="DigNum (strict)"("DisabledEnum"=w960) -> ()  [unwired: 2 in, 2 out]
        n607 = property on="3rd Point Cal" class="Bool (strict)"("DisabledEnum"=w960) -> ()  [unwired: 2 in, 2 out]
        n608 = property on="Reading Value 4" class="DigNum (strict)"("DisabledEnum"=w960) -> ()  [unwired: 2 in, 2 out]
        n609 = property on="Cal Value 4" class="DigNum (strict)"("DisabledEnum"=w960) -> ()  [unwired: 2 in, 2 out]
        n610 = property on="4th Point Cal" class="Bool (strict)"("DisabledEnum"=w960) -> ()  [unwired: 2 in, 2 out]
        n611 = property on="Reading Value 5" class="DigNum (strict)"("DisabledEnum"=w960) -> ()  [unwired: 2 in, 2 out]
        n612 = property on="Cal Value 5" class="DigNum (strict)"("DisabledEnum"=w960) -> ()  [unwired: 2 in, 2 out]
        n613 = property on="5th Point Cal" class="Bool (strict)"("DisabledEnum"=w960) -> ()  [unwired: 2 in, 2 out]
      }
      frame "Cal Review" {
        n614 = Unbundle By Name(w986) -> ("Auto"=w984:bool, "Verify Table"=w987:string[][])
        n615 = property on="Verify Table" class="Tbl (strict)"() -> ("EditPos"=w1000:T12)  [unwired: 2 in, 2 out]
        n616 = Unbundle(w1000) -> ("Row"=w998:i32)  [unwired: 1 out]
        n617 = local read "Ver Reading"() -> (w977:dbl)
        n618 = Greater Or Equal To 0?(x=w998) -> (x >= 0?=w999:bool)
        n619 = Index Array(array=w987, index (row)=w998, index (col)=0 ("disabled index (col)")) -> (element=w990:string)
        n620 = Fract/Exp String To Number(string=w990) -> (number=w979:dbl)  [unwired: 3 in, 1 out]
        n621 = case shown="True" w999 {
          tunnel: w998 -> [_ w1008]
          frame False {
          }
          frame True {
            "Row" <- w1008
          }
        }
        n622 = Increment(x=w977) -> (x+1=w991:dbl)
        n623 = Increment(x=w979) -> (x+1=w992:dbl)
        n624 = Subtract(x=w991, y=w992) -> (x-y=w980:dbl)
        n625 = Divide(x=w980, y=w991) -> (x/y=w996:dbl)
        n626 = local read "Lost Connection"() -> (w976:bool)
        n627 = Empty String/Path?(string/path=w990) -> (empty?=w983:bool)
        n628 = Absolute Value(x=w996) -> (abs(x)=w978:dbl)
        n629 = Not(x=w983) -> (.not. x?=w993:bool)
        n630 = Less?(x=w978, y=0.1) -> (x < y?=w994:bool)
        n631 = Compound Arithmetic op=AND(w984, w994, w993) -> (w989:bool)
        n632 = call "Reading Delay.vi"("Delay"="ms", "In Range"=w989) -> ("Take Reading"=w982:bool)  [unwired: 9 in]
        n633 = case shown="False" w976 {
          tunnel: [string[] ["Main", "Cal Review"] string[] ["End Cal"]] -> w1004
          frame False {
          }
          frame True {
          }
        }
        n634 = case shown="True" w982 {
          selector: w982 -> [_ w1007]
          frame False {
          }
          frame True {
            n635 = property on="Verify Read" class="Bool (strict)"("Val(Sgnl)"=w1007) -> ()  [unwired: 2 in, 2 out]
          }
        }
        n636 = Bundle By Name(cluster=w986, "Init Mean"=FALSE) -> (w981:T9)
        n637 = Insert Into Array(array=w1002, index=0, new element=w1004) -> (w1003:string[])
      }
      frame "Stop Verification" {
        w1009 = T10."Enabled" ("Disabled")
        n638 = property on="Header" class="Bool"("DisabledEnum"=w1009) -> ()  [unwired: 2 in, 2 out]
        n639 = property on="Channel to Cal" class="Enum (strict)"("DisabledEnum"=w1009) -> ()  [unwired: 2 in, 2 out]
        n640 = property on="View Spreadsheet" class="Bool"("DisabledEnum"=w1009) -> ()  [unwired: 2 in, 2 out]
        n641 = property on="Cal Unit" class="Enum (strict)"("DisabledEnum"=T10."Enabled" ("Disabled")) -> ()  [unwired: 2 in, 2 out]
        n642 = property on="Start Cal" class="Bool"("DisabledEnum"=w1009) -> ()  [unwired: 2 in, 2 out]
        n643 = disable-structure shown="Disabled" {
          disable-tunnel: w1009 -> [w1014 _]
          frame Disabled {
            n644 = property on="Start Verification" class="Bool"("DisabledEnum"=w1014) -> ()  [unwired: 2 in, 2 out]
          }
          frame Enabled {
          }
        }
        n645 = property on="Verify Tab" class="TabCtl (strict)"("Visible"=FALSE) -> ()  [unwired: 2 in, 2 out]
      }
      frame "Save Cal" {
        w1061 = u16 4 ("y")
        n646 = Unbundle By Name(w1036) -> ("Cal File Path"=w1046:path, "Cal Log Header"=w1068:string[], "Cal Log"=w1032:string[][], "Channel to Cal"=w1044:T1, "Cal Unit"=w1045:T2, "Verification"=w1035:bool, "Verify Table"=w1047:string[][])
        n647 = local read "Reading Value 1"() -> (w1029:dbl)
        n648 = local read "Reading Value 2"() -> (w1027:dbl)
        n649 = local read "Reading Value 3"() -> (w1025:dbl)
        n650 = local read "Reading Value 4"() -> (w1023:dbl)
        n651 = local read "Reading Value 5"() -> (w1021:dbl)
        n652 = local read "Cal Value 1"() -> (w1028:dbl)
        n653 = local read "Cal Value 2"() -> (w1026:dbl)
        n654 = local read "Cal Value 3"() -> (w1024:dbl)
        n655 = local read "Cal Value 4"() -> (w1022:dbl)
        n656 = local read "Cal Value 5"() -> (w1020:dbl)
        n657 = local read "a0"() -> (w1019:dbl)
        n658 = local read "a1"() -> (w1018:dbl)
        n659 = local read "a2"() -> (w1017:dbl)
        n660 = local read "a3"() -> (w1016:dbl)
        n661 = local read "a4"() -> (w1015:dbl)
        n662 = Build Array(w1029, w1028, w1027, w1026, w1025, w1024, w1023, w1022, w1021, w1020, w1019, w1018, w1017, w1016, w1015) -> (w1074:dbl[])
        n663 = Format Into String(w1044) -> (resulting string=w1040:string)  [unwired: 3 in, 1 out]
        n664 = Format Into String(w1045) -> (resulting string=w1037:string)  [unwired: 3 in, 1 out]
        n665 = Index Array(array=w1032, index (col) #1=0 ("disabled index (col)"), index (col) #2=1 ("index (col)")) -> (element #1=w1041:string[], element #2=w1039:string[])  [unwired: 2 in]
        n666 = Search 1D Array(1D array=w1041, element=w1040) -> (index of element=w1038:i32)  [unwired: 1 in]
        n667 = disable-structure shown="Disabled" {
          disable-tunnel: w1039 -> [w1081 _]
          disable-tunnel: w1038 -> [w1080 w1082]
          disable-tunnel: w1037 -> [w1079 _]
          disable-tunnel: [w1078 w1082] -> w1031
          frame Disabled {
            n668 = Search 1D Array(1D array=w1081, element=w1079, start index (0)=w1080) -> (index of element=w1078:i32)
          }
          frame Enabled {
          }
        }
        n669 = Index Array(array=w1047, index (col) #1=0 ("disabled index (col)"), index (col) #2=1 ("disabled index (col)")) -> (element #1=w1051:string[], element #2=w1050:string[])  [unwired: 2 in]
        n670 = Format Date/Time String(time format string (%c)="%d%b%y %I:%M:%S %p") -> (date/time string=w1072:string)  [unwired: 2 in]
        n671 = Interleave 1D Arrays(w1051, w1050) -> (w1049:string[])
        n672 = Index Array(array=w1032, index (row)=w1031) -> (element=w1030:string[])  [unwired: 1 in]
        n673 = To Upper Case(1:w1072) -> (0:w1034:string)
        n674 = case shown="False" w1035 {
          tunnel: w1074 -> [w1086 _]
          tunnel: [w1084 w1088] -> w1073
          tunnel: [w1083 w1087] -> w1033
          tunnel: w1034 -> [w1083 _]
          tunnel: w1030 -> [_ w1090]
          frame False {
            n675 = Number To Fractional String(number=w1086, precision (6)=i16 16) -> (F-format string=w1084:string[])  [unwired: 2 in]
          }
          frame True {
            n676 = Array Subset(array=w1090, index=2, length=9) -> (w1088:string[])
            n677 = Index Array(array=w1090, index=11) -> (element=w1087:string)
          }
        }
        n678 = Build Array (concatenate)(w1040, w1037, w1073, w1033, w1049) -> (w1070:string[])
        n679 = Greater?(x=w1031, y=w1061) -> (0:w1060:bool)
        n680 = Subtract(x=w1031, y=w1061) -> (x-y=w1059:i32)
        n681 = Bundle(cluster=T12 {"Row"=0, "Column"=0} ("Active Cell:Active Cell"), "Row"=w1031, "Column"=-2) -> (w1062:T12)
        n682 = Select(t=w1059, s=w1060, f=u16 0 ("y")) -> (s? t:f=w1056:i32)
        n683 = Replace Array Subset(array=w1032, new element=w1070, index (row)=w1031) -> (w1067:string[][])  [unwired: 1 in]
        n684 = Bundle(cluster=T12 {"Row"=0, "Column"=0} ("Active Cell:Active Cell"), "Row"=w1056, "Column"=0) -> (w1055:T12)
        n685 = Build Array (concatenate)(w1068, w1067) -> (w1066:string[][])
        n686 = Insert Into Array(array=w1075, index=0, new element=string[] ["Write to Excel", "Load Cal File", "End Cal", "Increment Channel"]) -> (w1076:string[])
        n687 = property on="Cal Table" class="Tbl (strict)"("Active Cell"=w1062, "Cell BG Color"=u32 16775793, "Index Values"=w1055) -> ()  [unwired: 2 in, 2 out]
        n688 = call-poly <vilib>:"Write To Spreadsheet File.vi"("delimiter (\\t)"="," ("delimiter (\\t)"), "2D data"=w1066, "file path (dialog if empty)"=w1046) -> ()  [unwired: 5 in, 1 out]
      }
      frame "Save Calibration" {
        w1139 = u16 4 ("y")
        n689 = Unbundle By Name(w1114) -> ("Cal File Path"=w1124:path, "Cal Log Header"=w1146:string[], "Cal Log"=w1110:string[][], "Channel to Cal"=w1122:T1, "Cal Unit"=w1123:T2, "Verification"=w1113:bool, "Verify Table"=w1125:string[][])
        n690 = local read "Reading Value 1"() -> (w1107:dbl)
        n691 = local read "Reading Value 2"() -> (w1105:dbl)
        n692 = local read "Reading Value 3"() -> (w1103:dbl)
        n693 = local read "Reading Value 4"() -> (w1101:dbl)
        n694 = local read "Reading Value 5"() -> (w1099:dbl)
        n695 = local read "Cal Value 1"() -> (w1106:dbl)
        n696 = local read "Cal Value 2"() -> (w1104:dbl)
        n697 = local read "Cal Value 3"() -> (w1102:dbl)
        n698 = local read "Cal Value 4"() -> (w1100:dbl)
        n699 = local read "Cal Value 5"() -> (w1098:dbl)
        n700 = local read "a0"() -> (w1097:dbl)
        n701 = local read "a1"() -> (w1096:dbl)
        n702 = local read "a2"() -> (w1095:dbl)
        n703 = local read "a3"() -> (w1094:dbl)
        n704 = local read "a4"() -> (w1093:dbl)
        n705 = Build Array(w1107, w1106, w1105, w1104, w1103, w1102, w1101, w1100, w1099, w1098, w1097, w1096, w1095, w1094, w1093) -> (w1152:dbl[])
        n706 = Format Into String(w1122) -> (resulting string=w1118:string)  [unwired: 3 in, 1 out]
        n707 = Format Into String(w1123) -> (resulting string=w1115:string)  [unwired: 3 in, 1 out]
        n708 = Index Array(array=w1110, index (col) #1=0 ("disabled index (col)"), index (col) #2=1 ("index (col)")) -> (element #1=w1119:string[], element #2=w1117:string[])  [unwired: 2 in]
        n709 = Search 1D Array(1D array=w1119, element=w1118) -> (index of element=w1116:i32)  [unwired: 1 in]
        n710 = disable-structure shown="Enabled" {
          disable-tunnel: w1117 -> [w1159 _]
          disable-tunnel: w1116 -> [w1158 w1160]
          disable-tunnel: w1115 -> [w1157 _]
          disable-tunnel: [w1156 w1160] -> w1109
          frame Disabled {
            n711 = Search 1D Array(1D array=w1159, element=w1157, start index (0)=w1158) -> (index of element=w1156:i32)
          }
          frame Enabled {
          }
        }
        n712 = Index Array(array=w1125, index (col) #1=0 ("disabled index (col)"), index (col) #2=1 ("disabled index (col)")) -> (element #1=w1129:string[], element #2=w1128:string[])  [unwired: 2 in]
        n713 = Format Date/Time String(time format string (%c)="%d%b%y %I:%M:%S %p") -> (date/time string=w1150:string)  [unwired: 2 in]
        n714 = Interleave 1D Arrays(w1129, w1128) -> (w1127:string[])
        n715 = Index Array(array=w1110, index (row)=w1109) -> (element=w1108:string[])  [unwired: 1 in]
        n716 = To Upper Case(1:w1150) -> (0:w1112:string)
        n717 = case shown="False" w1113 {
          tunnel: w1152 -> [w1164 _]
          tunnel: [w1162 w1166] -> w1151
          tunnel: [w1161 w1165] -> w1111
          tunnel: w1112 -> [w1161 _]
          tunnel: w1108 -> [_ w1168]
          frame False {
            n718 = Number To Fractional String(number=w1164, precision (6)=i16 16) -> (F-format string=w1162:string[])  [unwired: 2 in]
          }
          frame True {
            n719 = Array Subset(array=w1168, index=2, length=9) -> (w1166:string[])
            n720 = Index Array(array=w1168, index=11) -> (element=w1165:string)
          }
        }
        n721 = Build Array (concatenate)(w1118, w1115, w1151, w1111, w1127) -> (w1148:string[])
        n722 = Greater?(x=w1109, y=w1139) -> (0:w1138:bool)
        n723 = Subtract(x=w1109, y=w1139) -> (x-y=w1137:i32)
        n724 = Bundle(cluster=T12 {"Row"=0, "Column"=0} ("Active Cell:Active Cell"), "Row"=w1109, "Column"=-2) -> (w1140:T12)
        n725 = Select(t=w1137, s=w1138, f=u16 0 ("y")) -> (s? t:f=w1134:i32)
        n726 = Replace Array Subset(array=w1110, new element=w1148, index (row)=w1109) -> (w1145:string[][])  [unwired: 1 in]
        n727 = Bundle(cluster=T12 {"Row"=0, "Column"=0} ("Active Cell:Active Cell"), "Row"=w1134, "Column"=0) -> (w1133:T12)
        n728 = Build Array (concatenate)(w1146, w1145) -> (w1144:string[][])
        n729 = Insert Into Array(array=w1153, index=0, new element=string[] ["Write to Excel", "Load Cal File", "Cal Review Prep"]) -> (w1154:string[])
        n730 = property on="Cal Table" class="Tbl (strict)"("Active Cell"=w1140, "Cell BG Color"=u32 16775793, "Index Values"=w1133) -> ()  [unwired: 2 in, 2 out]
        n731 = call-poly <vilib>:"Write To Spreadsheet File.vi"("delimiter (\\t)"="," ("delimiter (\\t)"), "2D data"=w1144, "file path (dialog if empty)"=w1124) -> ()  [unwired: 5 in, 1 out]
      }
      frame "Distribute Calibration" {
        # "have to add in waiting screen, reread on main program, switch to streaming calibrated data and verification for that"
        n732 = Unbundle By Name(w1175) -> ("Desired System.ID"=w1172:string, "Cal File Path"=w1177:path)
        n733 = Concatenate Strings("10.30.189." ("string"), w1172) -> (w1173:string)
        n734 = Format Into String(format string="%s.cal", w1172) -> (resulting string=w1174:string)  [unwired: 2 in, 1 out]
        n735 = flat-sequence {
          tunnel: w1173 -> [w1183]
          tunnel: w1174 -> [w1182]
          tunnel: w1177 -> [w1181]
          frame #0 {
            n736 = call <vilib>:"FTP Put File.vi"("password"="", "user"="anonymous", "local path"=w1181, "remote path"=w1182, "host"=w1183) -> ()  [unwired: 5 in, 2 out]
          }
        }
      }
      frame "Calc Dev" {
        n737 = Unbundle By Name(w1191) -> ("Verify Table"=w1188:string[][], "Cal Unit"=w1186:T2, "Rack Version"=w1185:T5, "Verify Table Ref"=w1184:refnum<vi>)
        n738 = call "Calc Dev (DAQ Rack).vi"("Verify Table IN"=w1188, "Units"=w1186, "Rack Version"=w1185, "Dev Table 1 Ref"=w1184) -> ("Verify Table OUT"=w1187:string[][])  [unwired: 15 in]
        n739 = local write "Verify Table"(w1187) -> ()
        n740 = Bundle By Name(cluster=w1191, "Verify Table"=w1187) -> (w1190:T9)
        n741 = Insert Into Array(array=w1193, index=0, new element=string[] []) -> (w1192:string[])
      }
      frame "Write to Excel" {
        n742 = Unbundle By Name(w1202) -> ("Cal Spreadsheet Path"=w1206:path, "Verify Table"=w1199:string[][], "Channel to Cal"=w1196:T1, "Cal Unit"=w1195:T2)
        n743 = flat-sequence {
          tunnel: w1206 -> [w1213]
          tunnel: [w1213] -> w1207
          tunnel: [w1210] -> w1200
          tunnel: w1199 -> [w1210]
          tunnel: [w1209] -> w1198
          tunnel: w1196 -> [w1209]
          tunnel: [w1208] -> w1197
          tunnel: w1195 -> [w1208]
          tunnel: w1207 -> [w1217]
          tunnel: w1200 -> [w1216]
          tunnel: w1198 -> [w1215]
          tunnel: w1197 -> [w1214]
          frame #0 {
            n744 = property on="Main Tab" class="TabCtl (strict)"("DisabledEnum"=T10."Disabled" ("Disabled")) -> ()  [unwired: 2 in, 2 out]
            n745 = property on="Load Indicator Tab" class="TabCtl (strict)"("Visible"=TRUE) -> ()  [unwired: 2 in, 2 out]
          }
          frame #1 {
            n746 = call "Gas Rack Write Data.vi"("Cal Unit"=w1214, "Channel to Cal"=w1215, "Verify Table"=w1216, "Cal Path"=w1217) -> ()  [unwired: 8 in]
          }
          frame #2 {
            n747 = property on="Main Tab" class="TabCtl (strict)"("DisabledEnum"=T10."Enabled" ("Disabled")) -> ()  [unwired: 2 in, 2 out]
            n748 = property on="Load Indicator Tab" class="TabCtl (strict)"("Visible"=FALSE) -> ()  [unwired: 2 in, 2 out]
          }
        }
        n749 = Insert Into Array(array=w1204, index=0, new element=string[] ["Recolor Tables"]) -> (w1203:string[])
      }
      frame "Recolor Tables" {
        n750 = Unbundle By Name(w1224) -> ("Verify Table Ref"=w1223:refnum<vi>)
        n751 = property on="Property Node" class="Tbl (strict)"(reference=w1223, "Active Cell"=T12 {"Row"=-2, "Column"=-2} ("Active Cell:Active Cell"), "Cell BG Color"=u32 15527148) -> (reference out=w1220:refnum<vi>)  [unwired: 1 in, 1 out]
        n752 = property on="Property Node" class="Tbl (strict)"(reference=w1220, "Active Cell"=T12 {"Row"=-2, "Column"=1} ("Active Cell:Active Cell"), "Cell BG Color"=u32 16448250) -> ()  [unwired: 1 in, 2 out]
      }
      frame "End Cal" {
        w1228 = FALSE ("1st Point Cal")
        w1231 = T10."Disabled and Grayed Out" ("Disabled")
        w1233 = 0.0 ("Reading Value 1")
        w1237 = FALSE ("Visible")
        n753 = disable-structure shown="Disabled" {
          frame Disabled {
            n754 = property on="Cancel Verify" class="Bool"("Value"=FALSE ("Cancel Cal")) -> ()  [unwired: 2 in, 2 out]
          }
          frame Enabled {
          }
        }
        n755 = property on="Output Tab" class="TabCtl (strict)"("Visible"=w1237) -> ()  [unwired: 2 in, 2 out]
        n756 = property on="Header Tab" class="TabCtl (strict)"("Visible"=w1237) -> ()  [unwired: 2 in, 2 out]
        n757 = property on="Load Indicator Tab" class="TabCtl (strict)"("Visible"=w1237) -> ()  [unwired: 2 in, 2 out]
        n758 = property on="Main Tab" class="TabCtl (strict)"("DisabledEnum"=T10."Enabled" ("Disabled")) -> ()  [unwired: 2 in, 2 out]
        n759 = property on="Header" class="Bool"("DisabledEnum"=T10."Enabled" ("Disabled")) -> ()  [unwired: 2 in, 2 out]
        n760 = local write "Reading Value 1"(w1233) -> ()
        n761 = local write "Cal Value 1"(w1233) -> ()
        n762 = local write "Reading Value 2"(w1233) -> ()
        n763 = local write "Cal Value 2"(w1233) -> ()
        n764 = local write "Reading Value 3"(w1233) -> ()
        n765 = local write "Cal Value 3"(w1233) -> ()
        n766 = local write "Reading Value 4"(w1233) -> ()
        n767 = local write "Cal Value 4"(w1233) -> ()
        n768 = local write "Reading Value 5"(w1233) -> ()
        n769 = local write "Cal Value 5"(w1233) -> ()
        n770 = local write "a0"(w1233) -> ()
        n771 = local write "a1"(w1233) -> ()
        n772 = local write "a2"(w1233) -> ()
        n773 = local write "a3"(w1233) -> ()
        n774 = local write "a4"(w1233) -> ()
        n775 = property on="Start Cal" class="Bool"("DisabledEnum"=w1231) -> ()  [unwired: 2 in, 2 out]
        n776 = property on="Channel to Cal" class="Enum (strict)"("DisabledEnum"=w1231) -> ()  [unwired: 2 in, 2 out]
        n777 = property on="View Spreadsheet" class="Bool"("DisabledEnum"=w1231) -> ()  [unwired: 2 in, 2 out]
        n778 = property on="Start Verification" class="Bool"("DisabledEnum"=w1231) -> ()  [unwired: 2 in, 2 out]
        n779 = local write "Tank IP:"("" ("Tank IP:")) -> ()
        n780 = local write "RIO Found"(FALSE ("RIO Found")) -> ()
        n781 = call "TCP Data Stream PC.vi"("Mode"=TCP_Data_Stream_Mode_(PC)."Close") -> ()  [unwired: 15 in, 4 out]
        n782 = disable-structure shown="Disabled" {
          disable-tunnel: w1231 -> [w1242 _]
          frame Disabled {
            n783 = property on="Cal Unit" class="Enum (strict)"("DisabledEnum"=w1242) -> ()  [unwired: 2 in, 2 out]
          }
          frame Enabled {
          }
        }
        n784 = local write "1st Point Cal"(w1228) -> ()
        n785 = local write "2nd Point Cal"(w1228) -> ()
        n786 = local write "3rd Point Cal"(w1228) -> ()
        n787 = local write "4th Point Cal"(w1228) -> ()
        n788 = local write "5th Point Cal"(w1228) -> ()
        n789 = Insert Into Array(array=w1240, index=0, new element=string[] ["Recolor Tables", "Init Cal"]) -> (w1241:string[])
      }
      frame "Increment Channel" {
        n790 = Unbundle By Name(w1246) -> ("Channel to Cal"=w1245:T1)
        n791 = Increment(x=w1245) -> (x+1=w1244:T1)
        n792 = Bundle By Name(cluster=w1246, "Channel to Cal"=w1244) -> (w1247:T9)
        n793 = local write "Channel to Cal"(w1244) -> ()
      }
      frame "Exit" {
        n794 = local write "Stop Second Loop"(TRUE ("Stop Second Loop")) -> ()
      }
    }
  }
  n795 = while {
    tunnel: w2 -> [_]
    shift-right: [w1253] -> _
    shift-left: _ -> [w1254]
    stop <- "Stop Second Loop" stop-if-true
    n796 = local read "Channel to Cal"() -> (w1252:T1)
    n797 = local read "RIO Found"() -> (w1257:bool)
    n798 = Wait (ms)(milliseconds to wait=u32 10) -> ()  [unwired: 1 out]
    n799 = case shown="True" w1257 {
      tunnel: w1252 -> [_ w1262]
      tunnel: [0.0 ("Data Out") w1264] -> w1253
      tunnel: w1254 -> [_ w1263]
      frame False {
      }
      frame True {
        n800 = call "Gas Rack AI Read.vi"("Channel to Cal"=w1262) -> ("Lost Connection"=→"Lost Connection":bool, "Available?"=w1260:bool, "Data"=w1261:dbl)  [unwired: 8 in]
        n801 = case shown="False" w1260 {
          tunnel: w1261 -> [_ w1267]
          tunnel: [w1265 w1266] -> w1264
          tunnel: w1263 -> [w1265 _]
          frame False {
          }
          frame True {
            n802 = call <vilib>:"Mean PtByPt.vi"("x"=w1267, "sample length"="avg") -> ("mean"=w1266:dbl)  [unwired: 2 in, 1 out]
          }
        }
      }
    }
    "Cal Reading" <- w1253
    "Ver Reading" <- w1253
  }
  n803 = disable-structure shown="Disabled" {
    frame Disabled {
      n804 = property on="Verify Tab" class="TabCtl (strict)"("Visible"=TRUE) -> (error out=w1270:errorcluster)  [unwired: 2 in, 1 out]
      n805 = property on="Verify Table" class="Tbl (strict)"(error in=w1270, "Key Focus"=TRUE, "EditPos"=T12 {"Row"=0, "Column"=1} ("Active Cell:Active Cell")) -> ()  [unwired: 1 in, 2 out]
    }
    frame Enabled {
    }
  }
  n806 = disable-structure shown="Disabled" {
    frame Disabled {
      w1294 = 0 ("length")
      # "#Change In \"A\" selection added selection of \"RIO\" that links 25A Targets and Setpoints"
      n807 = Unbundle By Name() -> (w1290:T20, "Cal Targets Path"=w1283, "Targets"=w1288, "Cal Target Array"=w1304, "Channel to Cal"=w1305, "Verify Table"=w1277)
      n808 = property on="Cancel Verify" class="Bool"("DisabledEnum"=T10."Enabled" ("Disabled")) -> ()  [unwired: 2 in, 2 out]
      n809 = property on="Cal Table" class="Tbl (strict)"("Active Cell"=T12 {"Row"=-2, "Column"=-2} ("Active Cell:Active Cell"), "Cell BG Color"=u32 16448250) -> ()  [unwired: 2 in, 2 out]
      n810 = call <vilib>:"Open Config Data.vi"("configuration file path"=w1283) -> ("error out"=w1285:errorcluster, "refnum"=w1284:T15)  [unwired: 8 in, 1 out]
      n811 = call <userlib>:"Read INI Cluster__ogtk.vi"("error in (no error)"=w1285, "INI Fomatted Cluster Type"=w1288, "refnum"=w1284) -> ("error out"=w1287:errorcluster, "INI Fomatted Cluster"=w1289:variant, "dup refnum"=w1286:T15)  [unwired: 4 in, 2 out]
      n812 = Index Array(array=w1304, index=w1305) -> (element=w1300)
      n813 = call <vilib>:"Close Config Data.vi"("error in (no error)"=w1287, "refnum"=w1286) -> ()  [unwired: 8 in, 2 out]
      n814 = Variant To Data(type=w1288, Variant=w1289) -> (data=w1301)  [unwired: 1 in, 1 out]
      n815 = case shown="\"V\", Default" w1300 {
        tunnel: w1301 -> [w1310 w1313 w1316 w1319 w1322 w1325]
        tunnel: [w1308 w1311 w1314 w1317 w1320 w1323] -> w1303
        tunnel: [w1309 w1312 w1315 w1318 w1321 w1324] -> w1302
        frame "V", Default {
          n816 = Unbundle By Name(w1310) -> ("V Targets"=w1309, "V Setpoints"=w1308)
        }
        frame "A" {
          n817 = Unbundle By Name(w1313) -> ("A Targets"=w1312, "A Setpoints"=w1311)
        }
        frame "DegC" {
          n818 = Unbundle By Name(w1316) -> ("DegC Targets"=w1315, "DegC Setpoints"=w1314)
        }
        frame "kPa" {
          n819 = Unbundle By Name(w1319) -> ("kPa Targets"=w1318, "kPa Setpoints"=w1317)
        }
        frame "LpH" {
          n820 = Unbundle By Name(w1322) -> ("LpH Targets"=w1321, "LpH Setpoints"=w1320)
        }
        frame "CT" {
          n821 = Unbundle By Name(w1325) -> ("CT Targets"=w1324, "CT Setpoints"=w1323)
        }
      }
      n822 = Cluster To Array(cluster=w1302) -> (array=w1293:void[])
      n823 = Cluster To Array(cluster=w1303) -> (array=w1292:void[])
      n824 = Delete From Array(array=w1293, length=w1294, index=w1294) -> (deleted portion=w1298, array with subset deleted=w1295)
      n825 = call-poly <userlib>:"Remove Duplicates from 1D Array__ogtk.vi"("Input Array"=w1295) -> ("Output Array"=w1296:dbl[])  [unwired: 1 out]
      n826 = Build Array (concatenate)(w1298, w1296) -> (w1297:dbl[])
      n827 = Number To Fractional String(number=w1297, precision (6)=i16 3) -> (F-format string=w1291:string[])  [unwired: 2 in]
      n828 = Index Array(array=w1292) -> (element #1=w1280, element #2=w1281, element #3=w1282, element #4=w1306, element #5=w1307)  [unwired: 5 in]
      n829 = Replace Array Subset(array=w1277, new element=w1291, index (col)=0 ("disabled index (col)")) -> (w1279:string[])  [unwired: 1 in]
      n830 = local write "Cal Value 1"(w1280) -> ()
      n831 = local write "Cal Value 2"(w1281) -> ()
      n832 = local write "Cal Value 3"(w1282) -> ()
      n833 = local write "Cal Value 4"(w1306) -> ()
      n834 = local write "Cal Value 5"(w1307) -> ()
      n835 = Bundle By Name(cluster=w1290, "Targets"=w1301, "Verify Table"=w1279) -> (w1276:cluster{})
      n836 = property on="Verify Table" class="Tbl (strict)"("Value"=w1279) -> ()  [unwired: 2 in, 2 out]
    }
    frame Enabled {
    }
  }
